vi "main.vi"() -> ()   [LabVIEW 2013]
uses:
  measure/Meas Session.ctl
  adc/ADC Session.ctl
  drivers/niScope/niScope Session.ctl
  drivers/niScope/niScope Virtual Channel Config.ctl
  drivers/niScope/niScope Virtual Channel Mode.ctl
  drivers/niScope/niScope Virtual Channel Input Z.ctl
  drivers/niScope/niScope Virtual Channel Coupling.ctl
  drivers/niScope/niScope Type.ctl
  drivers/niScope/niScope Digitizing Process Options.ctl
  drivers/niScope/niScope Data Packet.ctl
  drivers/niScope/niScope Trigger Setup.ctl
  <instrlib>/niScope/Controls/niScope trigger coupling.ctl
  <instrlib>/niScope/Controls/niScope trigger slope.ctl
  drivers/DMM/3458A Digitizer Session.ctl
  drivers/DMM/3458A Virtual Channel Config.ctl
  drivers/Counter/Counter Session.ctl
  drivers/Counter/Counter Type.ctl
  drivers/AWG/AWG Session.ctl
  drivers/AWG/AWG Type.ctl
  drivers/DMM/3458A Sync Mode.ctl
  drivers/DMM/3458A Idn Mode.ctl
  drivers/DMM/3458A Digitizing Low Levels/Configure/Sampling Mode.ctl
  drivers/DMM/3458A Digitizing Process Options.ctl
  drivers/DMM/3458A Data Packet.ctl
  drivers/DMM/3458A Aux Record Data.ctl
  drivers/DMM/3458A Digitizing Low Levels/Configure/Level Setup.ctl
  drivers/DMM/3458A Digitizing Low Levels/Configure/First Sample Trigger.ctl
  drivers/DMM/3458A Aperture Selection Mode.ctl
  drivers/dsdll/DSDLL Session.ctl
  drivers/dsdll/dsdll.lvlibp/dsdll_instance.ctl
  drivers/dsdll/dsdll.lvlibp/dsdll_device_record.ctl
  drivers/dsdll/DSDLL Process Config.ctl
  drivers/dsdll/DSDLL Data Packet.ctl
  adc/ADC Type.ctl
  drivers/simulated_adc/SimAdc Config.ctl
  drivers/simulated_adc/SimAdc Channel Cfg.ctl
  adc/ADC On Close Action.ctl
  drivers/Quatsch_driver/QuADCDriver/QuADC Session.ctl
  drivers/Quatsch_driver/QuADCDriver/QuADC Virtual Channel Config.ctl
  drivers/Quatsch_driver/QuADCDriver/QuADC Virtual Channel Mode.ctl
  drivers/Quatsch_driver/QuADCDriver/QuADC Virtual Channel Input Z.ctl
  drivers/Quatsch_driver/QuADCDriver/QuADC Virtual Channel Coupling.ctl
  drivers/Quatsch_driver/QuADCDriver/QuADC Type.ctl
  drivers/Quatsch_driver/QuADCDriver/QuADC Digitizing Process Options.ctl
  drivers/Quatsch_driver/QuADCDriver/QuADC Data Packet.ctl
  drivers/Quatsch_driver/QuADCDriver/QuADC Trigger Setup.ctl
  measure/Meas Sequence Item.ctl
  measure/Meas Sampling Configuration.ctl
  adc/ADC Trig Config.ctl
  adc/ADC Trig Mode Source.ctl
  adc/ADC Trig Coupling.ctl
  adc/ADC Trig Slope.ctl
  measure/processing/QWTB/Meas Proc QWTB Algorithm Parameter Data.ctl
  measure/Meas Sequence Configuration.ctl
  measure/Meas Range Mode.ctl
  measure/Meas Sampling Rate Mode.ctl
  octave/golpi/mpc/golpi_session_ref.ctl
  octave/golpi/mpc/golpi_session.ctl
  octave/golpi/GOLPI Library.lvlibp/Public/GOLPI reference Type Def.ctl
  octave/golpi/GOLPI Library.lvlibp/LV Process source distribution/Pipe Handle.ctl
  measure/processing/Meas Process Config.ctl
  measure/processing/Meas Process Mode.ctl
  measure/processing/Meas Process Raw Config.ctl
  measure/processing/Meas Process Raw Result Mode.ctl
  measure/processing/QWTB/Meas Proc QWTB Setup.ctl
  measure/processing/QWTB/Meas Proc QWTB Uncertainty Mode.ctl
  measure/processing/QWTB/Meas Proc QWTB Multicore Setup.ctl
  measure/processing/QWTB/Meas Proc QWTB Multicore Type.ctl
  measure/Corrections/Corr Setup.ctl
  measure/Corrections/Corr Tranducer Item.ctl
  measure/Corrections/Corr Digitizers.ctl
  measure/Assist/Assist Panel Setup.ctl
  measure/processing/QWTB/Meas Proc QWTB View Max Dim.ctl
  measure/processing/QWTB/Meas Proc QWTB View Uncertainty Mode.ctl
  measure/processing/QWTB/Meas Proc QWTB View Group Mode.ctl
  measure/processing/QWTB/Meas Proc QWTB Viewer References.ctl
  measure/processing/QWTB/Meas Proc QWTB View Phase Mode.ctl
  server/Server Event GUI command.ctl
  server/Server Session.ctl
  varilib/SGUI Assign References Mode.ctl
  server/Server Event.ctl
  server/Server Client Request.ctl
  server/Server Event Command.ctl
  <vilib>/Utility/miscctls.llb/LVRowAndColumnTypeDef.ctl
  varilib/SGUI Assign Multiple Strings With Tags By Label.vi
  varilib/varilib.lvlib
  drivers/niScope/niScope Virtual Digitizer.lvlib
  drivers/DMM/3458A Virtual Digitizer.lvlib
  drivers/Counter/Counter.lvlib
  drivers/AWG/AWG.lvlib
  drivers/DMM/3458A Digitizing Low Levels/3458A Digitizing Low Levels.lvlib
  drivers/dsdll/DSDLL Virtual Digitizer.lvlib
  drivers/dsdll/dsdll.lvlibp
  octave/golpi/mpc/GOLPI Multi Process.lvlib
  drivers/Quatsch_driver/QuADCDriver/QuADC Virtual Digitizer.lvlib
  octave/golpi/GOLPI Library.lvlibp/LV Process source distribution/LV Process library.lvlib
  octave/golpi/GOLPI Library.lvlibp
panel:
  in  "btn view fft":bool
  in  "server":T1
  out "start btns":T2
  in  "server vi ref":refnum<vi>
  in  "btn srv":bool
  in  "btn qwtb calc":bool
  in  "qwtb view VI ref":refnum<vi>
  in  "exp tab":string[][](table)
  in  "btn about":bool
  out "qwtb view":T3
  in  "tc result":enum32{"RAW", "QWTB"}(tab)
  out "str res":string caption="Result"
  out "qwtb meas pth":string caption="Selected measurement:"
  in  "qwtb alg sel":u16(ring) caption="Algorithm selection"
  in  "qwtb meas sel":u16(ring) caption="Measurement selection" items=["None", "Current", "Load from file"]
  in  "qwtb ref chn":u16(ring) caption="Ref. channel" items=["None"]
  in  "qwtb ph unit":T4 caption="Phase mode"
  out "qwtb res info":string caption="Info:"
  in  "qwtb res sel":u16(ring) caption="Result selection" items=["Current result", "Average"]
  in  "qwtb maxarr":i32=10 caption="Max shown array size" min=1 max=1000 step=1
  in  "qwtb order":T5 caption="Res. order mode"
  in  "qwtb unc":T6 caption="Uncertainty display"
  in  "qwtb maxdim":T7 caption="Max. shown dimension"
  out "qwtb results table":string[][](table) caption="Results (right click to table to show actions)"
  in  "qwtb qu list":i32[](listbox) caption="Select quantities"
  in  "btn set&start":bool
  in  "btn setup":bool
  in  "btn corr":bool
  in  "btn view rec":bool
  in  "golpi":T8={"GOLPI ref"={"pipe handle"={"lv_proc.dll file path"=path "", "process instance handle"=[], "debug mode"=FALSE, "debug data"=[]}, "fast read timeout [ms]"=500, "fast read settle time [ms]"=10, "fast read to multiple [ms]"=1, "max elements per input line"=100, "slow read timeout [ms]"=5000, "stdin double format specifier"="%_16e", "max elements per stdout output column"=100, "console mode bitstream"=FALSE, "bitstream first read timeout [ms]"=1000, "bitstream read timeout [ms]"=50, "struct transfer possible"=FALSE, "matlab mode"=FALSE}, "idn str"="", "octave path"=path "C:/Octave364/Octave3.6.4_gcc4.6.2/bin", "work path"=path "C:/Octave364/Octave3.6.4_gcc4.6.2/bin", "start timeout [ms]"=15000, "clr cache"=FALSE, "console"=FALSE, "binary"=FALSE, "semaphore"=refnum, "initial command"="", "exit command"="", "matlab"=FALSE}
  out "stat3":string
  out "stat2":string
  in  "session VI ref":refnum<vi>
  out "stat1":string
  in  "session":T12={"adc"={"niScope"={"channel cfg"=[], "sessions"=[], "multi cards"=FALSE, "channels"=0, "type"=enum."n/a", "memory [B/chn]"=0, "ext. clock [Hz]"=0.0, "samples count"=0, "use streaming"=FALSE, "proc setup"={"packet size [smpl]"=0, "current timeout [s]"=0.0, "blk2blk timeout [s]"=0.0, "event time"=timestamp(0 s since 1904-01-01), "temp sampl T [s]"=0.0, "data queue"=refnum, "stop notifier"=refnum, "proc ref"=refnum}, "sample width [B]"=0, "ranges [V]"=[], "trigger setup"={"coupling"=1, "level [V]"=0.0, "slope"=0, "mode"=enum."Immediate"}, "fs [Hz]"=0.0, "bitres [bit]"=0}, "3458A"={"channels"=[], "sync unit"={"VISA"="", "type"=enum."Picotest U6200A"}, "awg unit"={"type"=enum."Agilent 331xxA to 332xxA", "VISA"="", "enable 10MHz ref"=FALSE}, "sync mode"=enum."MASTER-SLAVE, MASTER clocked by TIMER", "streaming mode"=FALSE, "idn mode"=enum."Auto", "sampling mode"=enum."DCV", "Ts [s]"=0.0, "sample memory [B]"=0, "proc setup"={"channel id"=0, "packet size [smpl]"=0, "current timeout [s]"=0.0, "blk2blk timeout [s]"=0.0, "event time"=timestamp(0 s since 1904-01-01), "stop notifier"=refnum, "data queues"=[], "proc refs"=[], "bus semaphore"=refnum}, "sample size [B]"=0, "sample count"=0, "aux data"={"channel id"=0, "valid?"=[], "gain [V]"=[], "timestamp [s]"=[], "Ts [s]"=0.0, "abs timestamp"=timestamp(0 s since 1904-01-01), "t [deg C]"=[]}, "ranges [V]"=[], "aperture [s]"=0.0, "LEVEL trigger"={"edge"=enum."POS", "level [V]"=0.0, "coupling"=enum."DC"}, "trigger mode"=enum."AUTO", "measure temp.?"=FALSE, "disp mesages"=[], "shared bus?"=FALSE, "disable display?"=FALSE, "aper mode"=enum."Manual", "aper rules"=[]}, "dsdll"={"dsdll"={"dsdll path"=path "", "dsdll handle"=[], "output devices"=[], "capture devices"=[]}, "channels"=0, "device id"=0, "channel idns"=[], "proc setup"={"packet size [smpl]"=0, "current timeout [s]"=0.0, "blk2blk timeout [s]"=0.0, "event time"=timestamp(0 s since 1904-01-01), "data queue"=refnum, "stop notifier"=refnum, "proc ref"=refnum}, "samples count"=0, "fs [Hz]"=0.0}, "type"=enum."niScope", "channel idn str"=[], "aux instr idn str"=[], "modified?"=FALSE, "simadc"={"channels"=[], "range [V]"=0.0, "Ts step [s]"=0.0, "time [s]"=0.0, "fs [Hz]"=0.0, "count"=0, "smpl offset"=0, "set count"=0, "bit res"=0}, "force rst?"=FALSE, "exit mode"=enum."Immediate reset", "exit dly"=0.0, "exit tmr"=timestamp(0 s since 1904-01-01), "busy?"=FALSE, "accessed?"=FALSE, "QuADC session"={"channel cfg"=[], "sessions"=[], "multi cards"=FALSE, "channels"=0, "type"=enum."n/a", "memory [B/chn]"=0, "ext. clock [Hz]"=0.0, "samples count"=0, "use streaming"=FALSE, "proc setup"={"packet size [smpl]"=0, "current timeout [s]"=0.0, "blk2blk timeout [s]"=0.0, "event time"=timestamp(0 s since 1904-01-01), "temp sampl T [s]"=0.0, "data queue"=refnum, "stop notifier"=refnum, "proc ref"=refnum}, "sample width [B]"=0, "ranges [V]"=[], "trigger setup"={"coupling"=1, "level [V]"=0.0, "slope"=0, "mode"=enum."Immediate"}, "fs [Hz]"=0.0, "bitres [bit]"=0}}, "sequence"=[], "sequence setup"={"group setups"=[], "average cycles"=0, "range mode"=enum."Keep defaults", "fs mode"=enum."Frequency", "rng even"=0.0, "rng odd"=0.0, "folder"=path "", "name base"="", "meas id"=0, "settle [s]"=0.0}, "golpi"=refnum, "processing setup"={"mode"=enum."Raw", "call after avgs?"=FALSE, "calculate?"=FALSE, "raw mode"={"command"="", "result mode"=enum."Display console output (only Octave)", "res variable"=""}, "QWTB"={"QWTB path"=path "", "alg filter path"="", "alg ids"=[], "alg parameters"=[], "parsed parameters"=[], "selected alg id"="", "selected unc mode"=enum."None", "qwtb mcc"=100, "qwtb timeout"=90, "qwtb covg"=95.0, "qwtb ofs"=0, "qwtb lim data"=0, "multicore"={"jobs folder"=path "", "cores"=0, "max jobs"=0, "mode"=enum."Singlecore"}, "unc once?"=FALSE}}, "corrections"={"transducers"={"channels"=[], "last path"=path ""}, "digitizer"={"last path"=path "", "channel paths"=[], "channel idns"=[], "correction name"="", "channel names"=[], "folders to copy"=[], "channel valid"=[], "correction path"=path "", "correction rel path"="", "rel folders to copy"=[]}}, "assist cfg"={"P"=0, "Q"=0, "rel shift"=0.0, "ref freq"=0.0, "min fs"=0.0, "max fs tol"=0.0, "min int"=0.0, "max int"=0.0, "max err"=0.0, "max timeout"=0.0}} {"corrections"."transducers"."channels"."Phase index" min=1 step=1; "adc"."QuADC session"."trigger setup"."level [V]" format="%.2f"; "adc"."QuADC session"."trigger setup"."coupling" items=["AC"=0, "DC"=1, "HF Reject"=3, "LF Reject"=4, "AC Plus HF Reject"=1001]; "adc"."QuADC session"."channel cfg"."Clock fr. (Hz)" min=0.0 format="%#_9p"; "adc"."QuADC session"."channel cfg"."Number of JJ" min=1; "adc"."QuADC session"."channel cfg"."Range [Vpk]" min=0.0; "adc"."QuADC session"."channel cfg"."Channel" min=0; "adc"."3458A"."channels"."Range [Vpk]" min=0.0; "adc"."niScope"."trigger setup"."level [V]" format="%.2f"; "adc"."niScope"."trigger setup"."coupling" items=["AC"=0, "DC"=1, "HF Reject"=3, "LF Reject"=4, "AC Plus HF Reject"=1001]; "adc"."niScope"."channel cfg"."Range [Vpk]" min=0.0; "adc"."niScope"."channel cfg"."Channel" min=0}
  in  "btn stop":bool
  in  "btn start":bool
  out "error":errorcluster
  in  "btn exit":bool
  in  "btn cfg adc":bool
  in  "btn cfg octave":bool
  # "ADC:"
  # "IP Address"
  # "."
  # "."
  # "."
  # ":"
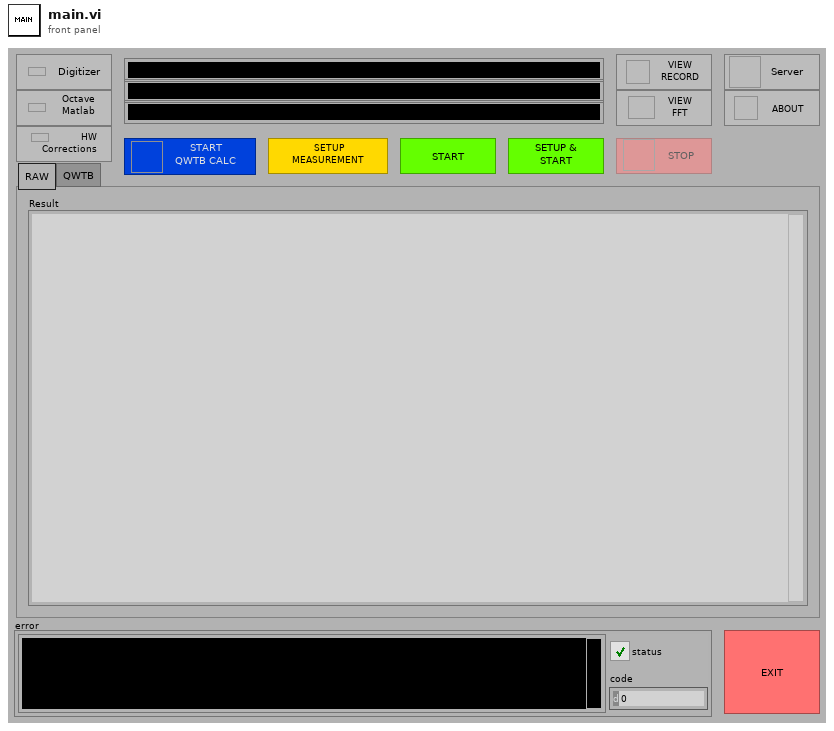
[diagram p1: front panel]
types:
  T1 = typedef "Server Session.ctl" = cluster{"cmd event":variant, "answer event":variant}
  T2 = typedef "Server Event GUI command.ctl" = cluster{"start":bool, "setup":bool, "setup&start":bool}
  T3 = typedef "Meas Proc QWTB Viewer References.ctl" = cluster{"tc result":refnum<vi>, "qwtb results tbl":refnum<vi>, "qwtb maxdim":refnum<vi>, "qwtb unc":refnum<vi>, "qwtb order":refnum<vi>, "qwtb maxarr":refnum<vi>, "qwtb res sel":refnum<vi>, "qwtb res info":refnum<vi>, "descriptions":string[], "var names":string[], "channel indexes":i32[], "qwtb ref chn":refnum<vi>, "qwtb ph unit":refnum<vi>, "qwtb alg sel":refnum<vi>, "qwtb meas sel":refnum<vi>, "qwtb ssn info":refnum<vi>, "last session":path, "qwtb qu list":refnum<vi>}
  T4 = typedef "Meas Proc QWTB View Phase Mode.ctl" = enum16{"± pi [rad]", "0 - 2*pi [rad]", "±180 [deg]", "0 - 360 [deg]"}
  T5 = typedef "Meas Proc QWTB View Group Mode.ctl" = enum16{"Group quantities", "Group phases"}
  T6 = typedef "Meas Proc QWTB View Uncertainty Mode.ctl" = enum16{"None", "val ± unc", "[val; unc]"}
  T7 = typedef "Meas Proc QWTB View Max Dim.ctl" = enum16{"Scalar", "Vector", "Matrix"}
  T8 = typedef "GOLPI Multi Process.lvlib/golpi_session.ctl" = cluster{"GOLPI ref":T9, "idn str":string, "octave path":path, "work path":path, "start timeout [ms]":u32, "clr cache":bool, "console":bool, "binary":bool, "semaphore":T11, "initial command":string, "exit command":string, "matlab":bool}
  T9 = typedef "GOLPI Library.lvlibp/GOLPI reference Type Def.ctl" = cluster{"pipe handle":T10, "fast read timeout [ms]":u32, "fast read settle time [ms]":u32, "fast read to multiple [ms]":u32, "max elements per input line":u32, "slow read timeout [ms]":u32, "stdin double format specifier":string, "max elements per stdout output column":u32, "console mode bitstream":bool, "bitstream first read timeout [ms]":u32, "bitstream read timeout [ms]":u32, "struct transfer possible":bool, "matlab mode":bool}
  T10 = typedef "GOLPI Library.lvlibp/LV Process library.lvlib/Pipe Handle.ctl" = cluster{"lv_proc.dll file path":path, "process instance handle":u32[], "debug mode":bool, "debug data":cluster{"time":timestamp, "stdin":bool, "data":string}[]}
  T11 = typedef "Semaphore RefNum" = refnum<k1>
  T12 = typedef "Meas Session.ctl" = cluster{"adc":T13, "sequence":T54[], "sequence setup":T61, "golpi":T64, "processing setup":T65, "corrections":T73, "assist cfg":T76}
  T13 = typedef "ADC Session.ctl" = cluster{"niScope":T14, "3458A":T24, "dsdll":T38, "type":T42, "channel idn str":string[], "aux instr idn str":string[], "modified?":bool, "simadc":T43, "force rst?":bool, "exit mode":T45, "exit dly":dbl, "exit tmr":timestamp, "busy?":bool, "accessed?":bool, "QuADC session":T46}
  T14 = typedef "niScope Virtual Digitizer.lvlib/niScope Session.ctl" = cluster{"channel cfg":T15[], "sessions":refnum<k20>[], "multi cards":bool, "channels":i32, "type":T19, "memory [B/chn]":i32, "ext. clock [Hz]":dbl, "samples count":i64, "use streaming":bool, "proc setup":T20, "sample width [B]":i32, "ranges [V]":dbl[], "trigger setup":T21, "fs [Hz]":dbl, "bitres [bit]":i32}
  T15 = typedef "niScope Virtual Digitizer.lvlib/niScope Virtual Channel Config.ctl" = cluster{"Address":refnum<k15>, "Channel":i32, "Mode":T16, "Input Z":T17, "Coupling":T18, "Range [Vpk]":dbl, "btn clr":bool, "btn up":bool, "btn down":bool}
  T16 = typedef "niScope Virtual Digitizer.lvlib/niScope Virtual Channel Mode.ctl" = enum16{"Single ended", "Unbal. differential", "Differential"}
  T17 = typedef "niScope Virtual Digitizer.lvlib/niScope Virtual Channel Input Z.ctl" = enum16{"1 MOhm", "50 Ohm"}
  T18 = typedef "niScope Virtual Digitizer.lvlib/niScope Virtual Channel Coupling.ctl" = enum16{"AC", "DC", "GND"}
  T19 = typedef "niScope Virtual Digitizer.lvlib/niScope Type.ctl" = enum16{"n/a", "5922"}
  T20 = typedef "niScope Virtual Digitizer.lvlib/niScope Digitizing Process Options.ctl" = cluster{"packet size [smpl]":i64, "current timeout [s]":dbl, "blk2blk timeout [s]":dbl, "event time":timestamp, "temp sampl T [s]":dbl, "data queue":refnum<queue>, "stop notifier":refnum<notifier>, "proc ref":refnum<vi>}
  T21 = typedef "niScope Virtual Digitizer.lvlib/niScope Trigger Setup.ctl" = cluster{"coupling":T22, "level [V]":dbl, "slope":T23, "mode":enum16{"Immediate", "External", "Level"}}
  T22 = typedef "niScope trigger coupling.ctl" = u16
  T23 = typedef "niScope trigger slope.ctl" = i32
  T24 = typedef "3458A Virtual Digitizer.lvlib/3458A Digitizer Session.ctl" = cluster{"channels":T25[], "sync unit":T26, "awg unit":T28, "sync mode":T30, "streaming mode":bool, "idn mode":T31, "sampling mode":T32, "Ts [s]":dbl, "sample memory [B]":i32, "proc setup":T33, "sample size [B]":i32, "sample count":i32, "aux data":T34, "ranges [V]":dbl[], "aperture [s]":dbl, "LEVEL trigger":T35, "trigger mode":T36, "measure temp.?":bool, "disp mesages":string[], "shared bus?":bool, "disable display?":bool, "aper mode":T37, "aper rules":dbl[][]}
  T25 = typedef "3458A Virtual Digitizer.lvlib/3458A Virtual Channel Config.ctl" = cluster{"VISA":refnum<visa-resource-name>, "Range [Vpk]":dbl, "btn clr":bool, "btn up":bool, "btn down":bool}
  T26 = typedef "Counter.lvlib/Counter Session.ctl" = cluster{"VISA":refnum<visa-resource-name>, "type":T27}
  T27 = typedef "Counter.lvlib/Counter Type.ctl" = enum16{"Picotest U6200A", "dummy"}
  T28 = typedef "AWG.lvlib/AWG Session.ctl" = cluster{"type":T29, "VISA":refnum<visa-resource-name>, "enable 10MHz ref":bool}
  T29 = typedef "AWG.lvlib/AWG Type.ctl" = enum16{"Agilent 331xxA to 332xxA", "Agilent 335xxA to 336xxA", "Tektronix AFG3101C", "dummy"}
  T30 = typedef "3458A Virtual Digitizer.lvlib/3458A Sync Mode.ctl" = enum16{"MASTER-SLAVE, MASTER clocked by TIMER", "MASTER-SLAVE, MASTER clocked by AWG", "ALL clocked by AWG", "MASTER-SLAVE, ALL clocked by TIMER", "ALL clocked by AWG with DFLL"}
  T31 = typedef "3458A Virtual Digitizer.lvlib/3458A Idn Mode.ctl" = enum16{"Auto", "Sequential (chn A, chn B, ...)", "From calibration string"}
  T32 = typedef "3458A Virtual Digitizer.lvlib/3458A Digitizing Low Levels.lvlib/Sampling Mode.ctl" = enum16{"DCV", "DSDC", "DSAC"}
  T33 = typedef "3458A Virtual Digitizer.lvlib/3458A Digitizing Process Options.ctl" = cluster{"channel id":i32, "packet size [smpl]":i32, "current timeout [s]":dbl, "blk2blk timeout [s]":dbl, "event time":timestamp, "stop notifier":refnum<notifier>, "data queues":refnum<queue>[], "proc refs":refnum<vi>[], "bus semaphore":T11}
  T34 = typedef "3458A Virtual Digitizer.lvlib/3458A Aux Record Data.ctl" = cluster{"channel id":i32, "valid?":bool[], "gain [V]":dbl[], "timestamp [s]":dbl[], "Ts [s]":dbl, "abs timestamp":timestamp, "t [deg C]":dbl[]}
  T35 = typedef "3458A Virtual Digitizer.lvlib/3458A Digitizing Low Levels.lvlib/Level Setup.ctl" = cluster{"edge":enum16{"POS", "NEG"}, "level [V]":dbl, "coupling":enum16{"DC", "AC"}}
  T36 = typedef "3458A Virtual Digitizer.lvlib/3458A Digitizing Low Levels.lvlib/First Sample Trigger.ctl" = enum16{"AUTO", "EXT", "SYN", "SGL", "HOLD", "LEVEL"}
  T37 = typedef "3458A Virtual Digitizer.lvlib/3458A Aperture Selection Mode.ctl" = enum16{"Manual", "Maximum", "Table"}
  T38 = typedef "DSDLL Virtual Digitizer.lvlib/DSDLL Session.ctl" = cluster{"dsdll":T39, "channels":i32, "device id":i32, "channel idns":string[], "proc setup":T41, "samples count":i32, "fs [Hz]":dbl}
  T39 = typedef "dsdll.lvlibp/dsdll_instance.ctl" = cluster{"dsdll path":path, "dsdll handle":u8[], "output devices":T40[], "capture devices":T40[]}
  T40 = typedef "dsdll.lvlibp/dsdll_device_record.ctl" = cluster{"guid":u8[], "name":string}
  T41 = typedef "DSDLL Virtual Digitizer.lvlib/DSDLL Process Config.ctl" = cluster{"packet size [smpl]":i32, "current timeout [s]":dbl, "blk2blk timeout [s]":dbl, "event time":timestamp, "data queue":refnum<queue>, "stop notifier":refnum<notifier>, "proc ref":refnum<vi>}
  T42 = typedef "ADC Type.ctl" = enum16{"niScope", "3458A", "DirectSound DLL", "dummy", "QuADC"}
  T43 = typedef "SimAdc Config.ctl" = cluster{"channels":T44[], "range [V]":dbl, "Ts step [s]":dbl, "time [s]":dbl, "fs [Hz]":dbl, "count":i64, "smpl offset":i64, "set count":i64, "bit res":i32}
  T44 = typedef "SimAdc Channel Cfg.ctl" = cluster{"harmonics":dbl[][], "btn clear":bool, "noise":dbl, "fundamental [Hz]":dbl}
  T45 = typedef "ADC On Close Action.ctl" = enum16{"Immediate reset", "Delayed reset"}
  T46 = typedef "QuADC Virtual Digitizer.lvlib/QuADC Session.ctl" = cluster{"channel cfg":T47[], "sessions":refnum<k5>[], "multi cards":bool, "channels":i32, "type":T51, "memory [B/chn]":i32, "ext. clock [Hz]":dbl, "samples count":i64, "use streaming":bool, "proc setup":T52, "sample width [B]":i32, "ranges [V]":dbl[], "trigger setup":T53, "fs [Hz]":dbl, "bitres [bit]":i32}
  T47 = typedef "QuADC Virtual Digitizer.lvlib/QuADC Virtual Channel Config.ctl" = cluster{"Channel":i32, "Mode":T48, "Input Z":T49, "Coupling":T50, "Range [Vpk]":dbl, "btn clr":bool, "btn up":bool, "btn down":bool, "IP address A":u8, "IP address B":u8, "IP address C":u8, "IP address D":u8, "Port":u16, "Number of JJ":u32, "Clock fr. (Hz)":dbl}
  T48 = typedef "QuADC Virtual Digitizer.lvlib/QuADC Virtual Channel Mode.ctl" = enum16{"Single ended", "Unbal. differential", "Differential"}
  T49 = typedef "QuADC Virtual Digitizer.lvlib/QuADC Virtual Channel Input Z.ctl" = enum16{"1 MOhm", "50 Ohm"}
  T50 = typedef "QuADC Virtual Digitizer.lvlib/QuADC Virtual Channel Coupling.ctl" = enum16{"AC", "DC", "GND"}
  T51 = typedef "QuADC Virtual Digitizer.lvlib/QuADC Type.ctl" = enum16{"n/a", "v1"}
  T52 = typedef "QuADC Virtual Digitizer.lvlib/QuADC Digitizing Process Options.ctl" = cluster{"packet size [smpl]":i64, "current timeout [s]":dbl, "blk2blk timeout [s]":dbl, "event time":timestamp, "temp sampl T [s]":dbl, "data queue":refnum<queue>, "stop notifier":refnum<notifier>, "proc ref":refnum<vi>}
  T53 = typedef "QuADC Virtual Digitizer.lvlib/QuADC Trigger Setup.ctl" = cluster{"coupling":T22, "level [V]":dbl, "slope":T23, "mode":enum16{"Immediate", "External", "Level"}}
  T54 = typedef "Meas Sequence Item.ctl" = cluster{"config":T55, "data file path":path, "header file path":path, "group id":i32, "average id":i32, "group done?":bool, "adc modified?":bool, "source modified?":bool, "progress [%]":dbl, "groups cnt":i32, "average cnt":i32, "data file relative path":string, "meas root path":path, "calculate?":bool}
  T55 = typedef "Meas Sampling Configuration.ctl" = cluster{"fs [Hz]":dbl, "count [smpl]":i64, "aperture [s]":dbl, "trigger":T56, "ranges [Vpk]":dbl[], "QWTB parameters":T60[]}
  T56 = typedef "ADC Trig Config.ctl" = cluster{"source":T57, "level [V]":dbl, "coupling":T58, "slope":T59}
  T57 = typedef "ADC Trig Mode Source.ctl" = enum16{"Immediate", "External", "Level"}
  T58 = typedef "ADC Trig Coupling.ctl" = enum16{"DC", "AC"}
  T59 = typedef "ADC Trig Slope.ctl" = enum16{"POS", "NEG"}
  T60 = typedef "Meas Proc QWTB Algorithm Parameter Data.ctl" = cluster{"name":string, "numerics":dbl[], "strings":string[]}
  T61 = typedef "Meas Sequence Configuration.ctl" = cluster{"group setups":T55[], "average cycles":i32, "range mode":T62, "fs mode":T63, "rng even":dbl, "rng odd":dbl, "folder":path, "name base":string, "meas id":i32, "settle [s]":dbl}
  T62 = typedef "Meas Range Mode.ctl" = enum16{"Keep defaults", "Set All channels", "Set Odd and Even channels"}
  T63 = typedef "Meas Sampling Rate Mode.ctl" = enum16{"Frequency", "Period"}
  T64 = typedef "GOLPI Multi Process.lvlib/golpi_session_ref.ctl" = refnum<vi>
  T65 = typedef "Meas Process Config.ctl" = cluster{"mode":T66, "call after avgs?":bool, "calculate?":bool, "raw mode":T67, "QWTB":T69}
  T66 = typedef "Meas Process Mode.ctl" = enum16{"Raw", "QWTB"}
  T67 = typedef "Meas Process Raw Config.ctl" = cluster{"command":string, "result mode":T68, "res variable":string}
  T68 = typedef "Meas Process Raw Result Mode.ctl" = enum16{"Display console output (only Octave)", "Display string variable", "Display result file %respath%"}
  T69 = typedef "Meas Proc QWTB Setup.ctl" = cluster{"QWTB path":path, "alg filter path":string, "alg ids":string[], "alg parameters":string[], "parsed parameters":T60[], "selected alg id":string, "selected unc mode":T70, "qwtb mcc":i32, "qwtb timeout":i32, "qwtb covg":dbl, "qwtb ofs":i64, "qwtb lim data":i64, "multicore":T71, "unc once?":bool}
  T70 = typedef "Meas Proc QWTB Uncertainty Mode.ctl" = enum16{"None", "GUF", "Monte Carlo"}
  T71 = typedef "Meas Proc QWTB Multicore Setup.ctl" = cluster{"jobs folder":path, "cores":i32, "max jobs":i32, "mode":T72}
  T72 = typedef "Meas Proc QWTB Multicore Type.ctl" = enum16{"Singlecore", "Multicore", "Multistation"}
  T73 = typedef "Corr Setup.ctl" = cluster{"transducers":cluster{"channels":T74[], "last path":path}, "digitizer":T75}
  T74 = typedef "Corr Tranducer Item.ctl" = cluster{"Path":path, "Ratio:":string, "Name:":string, "btn rem":bool, "btn up":bool, "btn down":bool, "s.n.:":string, "btn open":bool, "ratio o/i":dbl, "chn hi":u16, "chn lo":u16, "Phase index":i32}
  T75 = typedef "Corr Digitizers.ctl" = cluster{"last path":path, "channel paths":path[], "channel idns":string[], "correction name":string, "channel names":string[], "folders to copy":path[], "channel valid":bool[], "correction path":path, "correction rel path":string, "rel folders to copy":string[]}
  T76 = typedef "Assist Panel Setup.ctl" = cluster{"P":i32, "Q":i32, "rel shift":dbl, "ref freq":dbl, "min fs":dbl, "max fs tol":dbl, "min int":dbl, "max int":dbl, "max err":dbl, "max timeout":dbl}
  T77 = typedef "varilib.lvlib/SGUI Assign References Mode.ctl" = enum16{"Add to stack", "Overwrite", "Release last", "Release ID"}
  T78 = typedef "Server Event Command.ctl" = enum16{"None", "Restart", "Identify", "Set measurement", "Start", "Get status", "Get result", "Stop", "Set corrections", "Get algorithm info"}
  T79 = typedef "Server Event.ctl" = cluster{"client request":T80, "command":T78}
  T80 = typedef "Server Client Request.ctl" = cluster{"info data":string, "answer handle":i32}
  T81 = enum8{"Enabled", "Disabled", "Disabled and Grayed Out"}
  T82 = typedef "Meas Proc QWTB Plot Config.ctl" = cluster{"X-axis style":T83, "Y-axis style":T83, "Show legend":T84, "Grid on":bool, "Box on":bool, "show all chn":bool}
  T83 = typedef "Meas Proc QWTB Plot Scale Mode.ctl" = enum16{"Linear", "Log"}
  T84 = typedef "Meas Proc QWTB Plot Legend.ctl" = enum16{"None", "Best", "North", "South", "East", "West", "NorthEast", "NorthWest", "SouthEast", "SouthWest"}
  T85 = typedef "LVRowAndColumnTypeDef.ctl" = cluster{"Row":i32, "Column":i32}
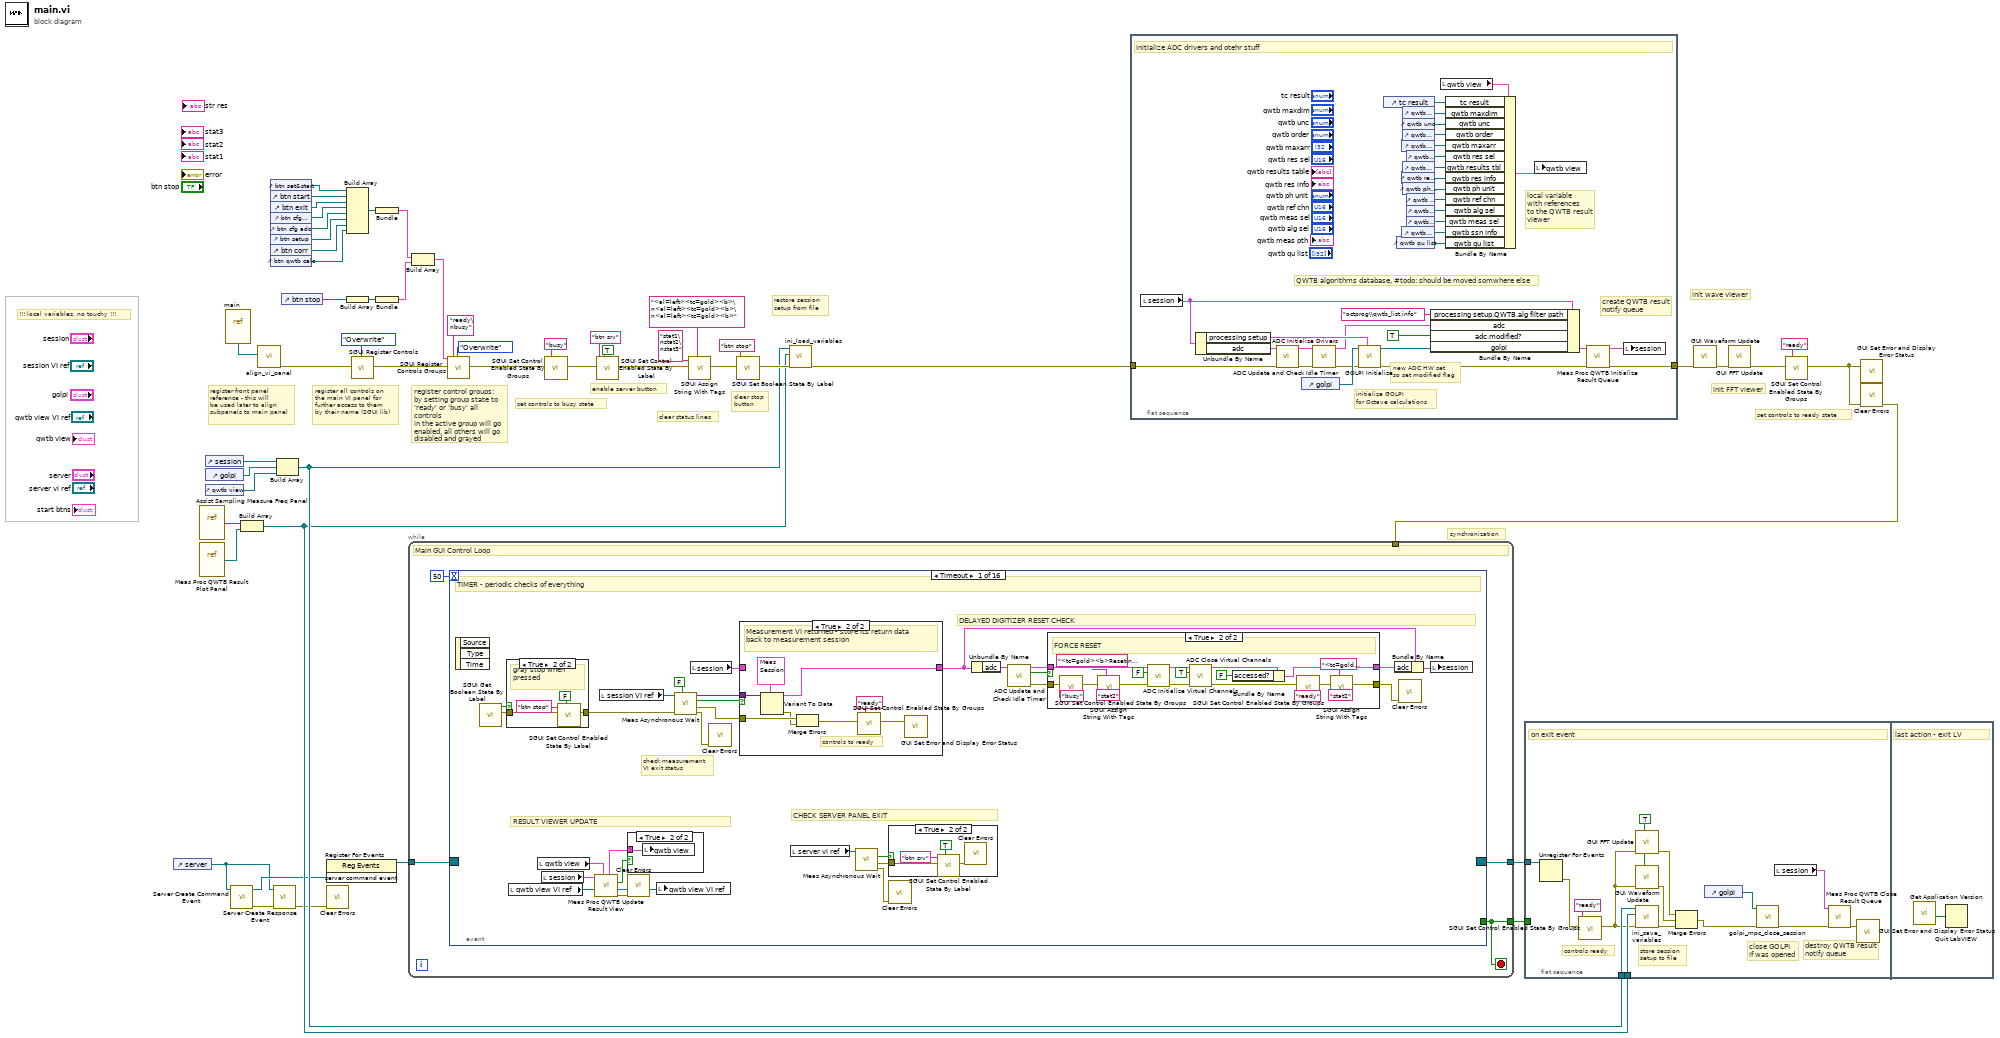
[diagram p0: block diagram]
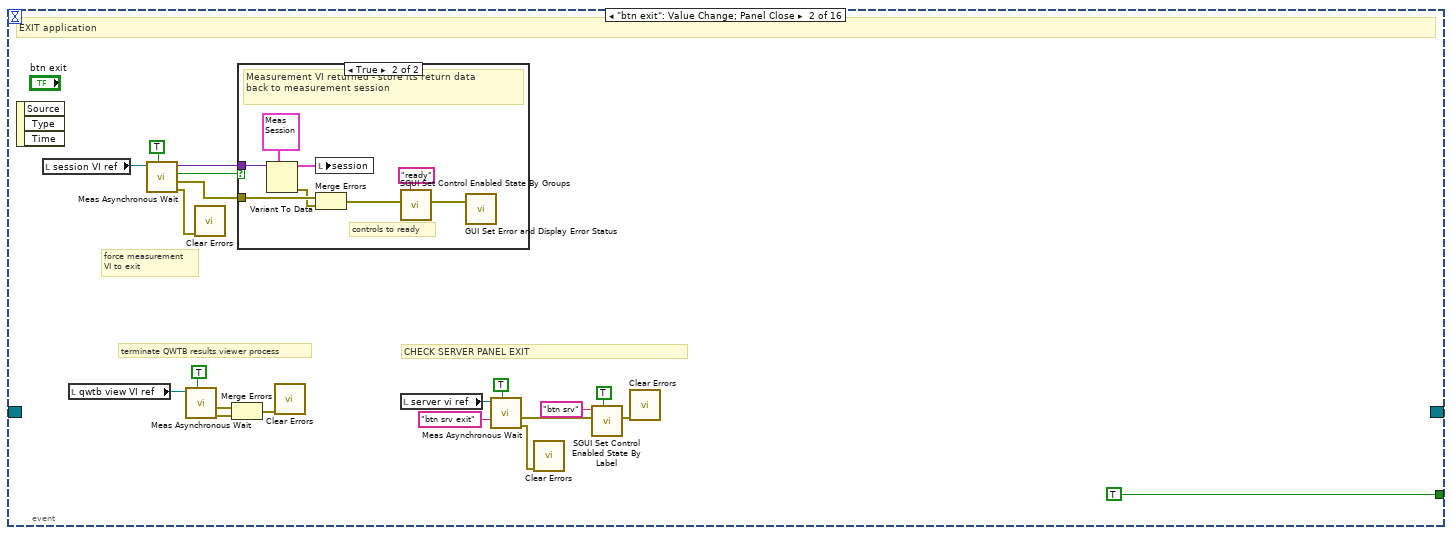
[diagram p7: hidden frame]
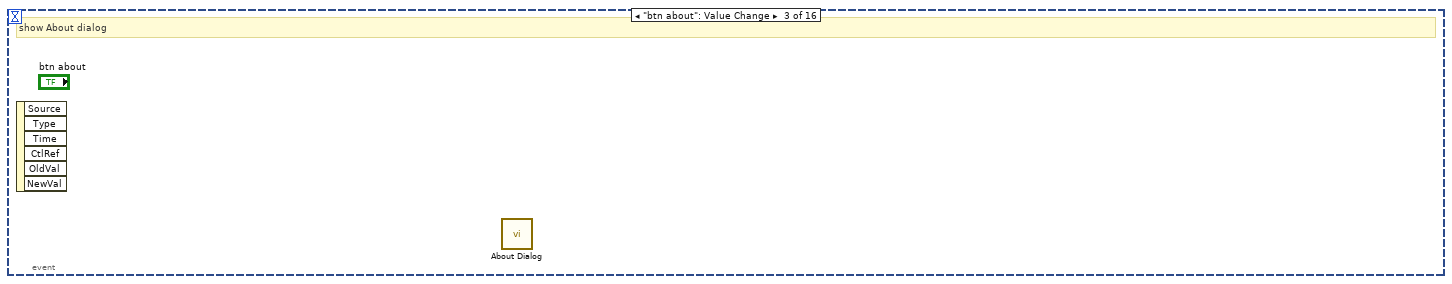
[diagram p9: hidden frame]
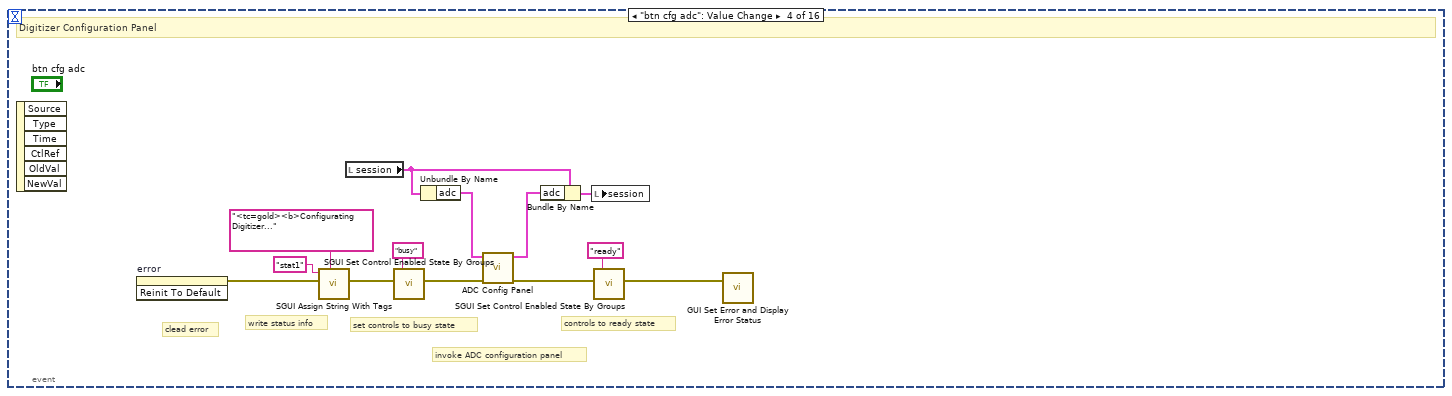
[diagram p10: hidden frame]
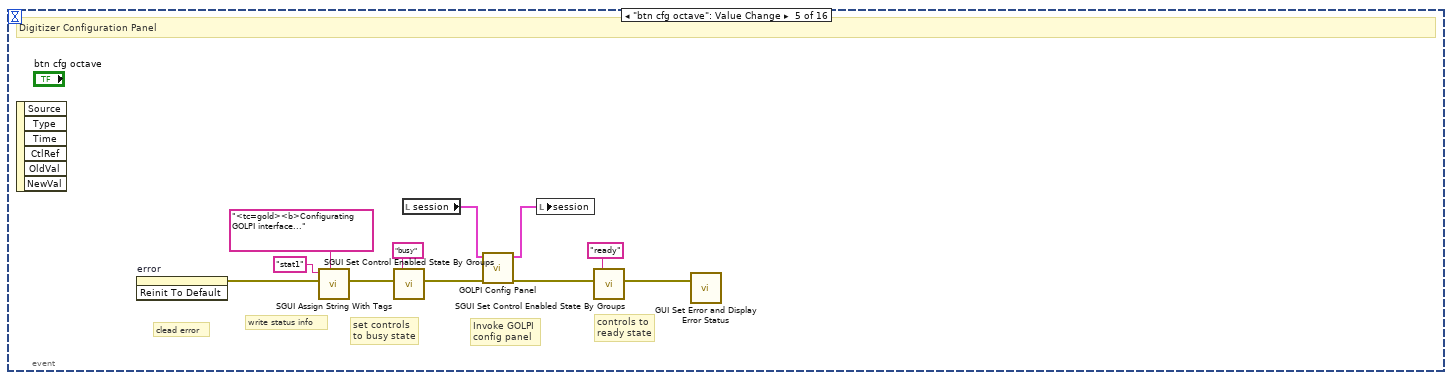
[diagram p11: hidden frame]
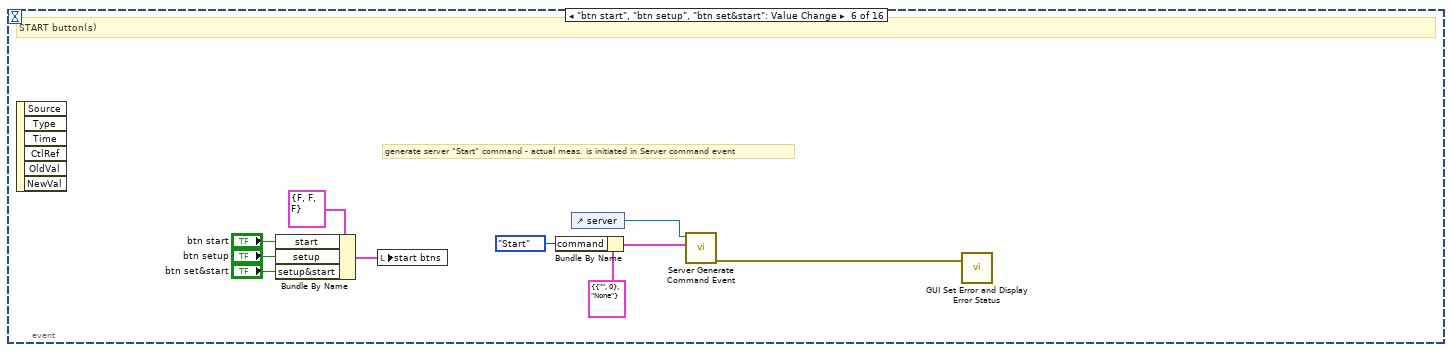
[diagram p12: hidden frame]
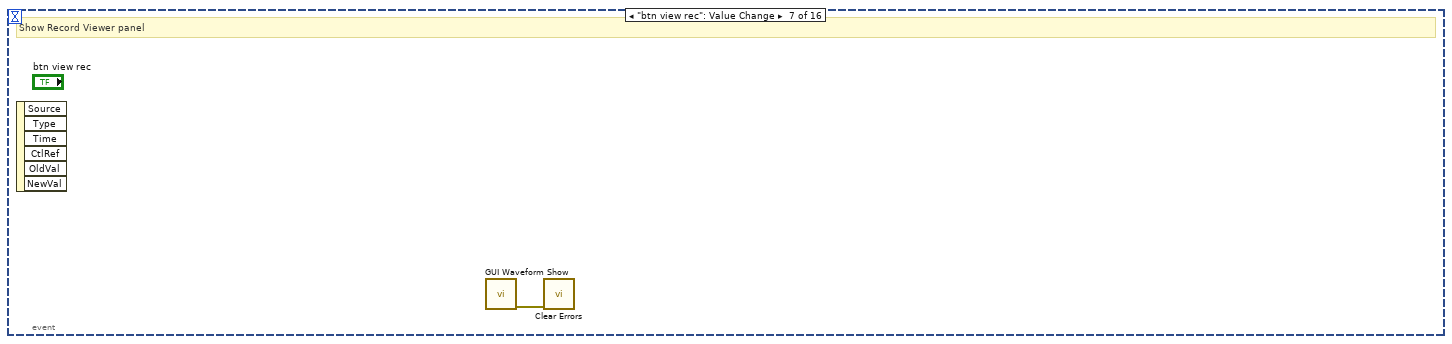
[diagram p13: hidden frame]
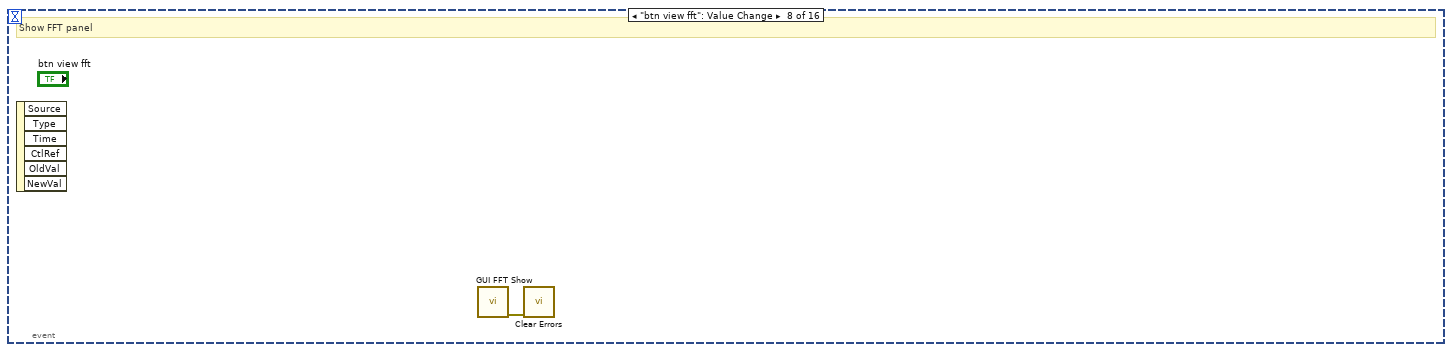
[diagram p14: hidden frame]
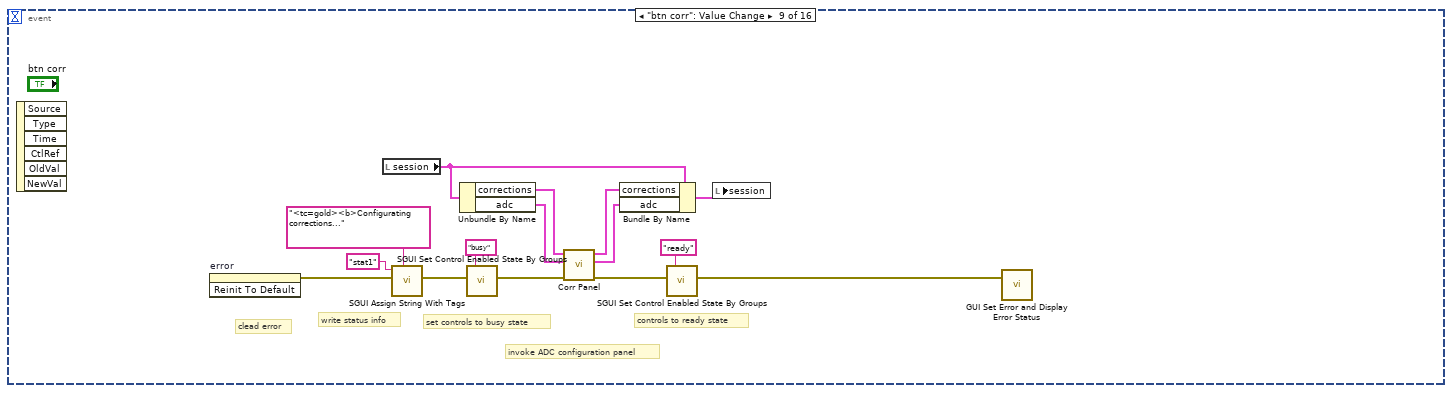
[diagram p15: hidden frame]
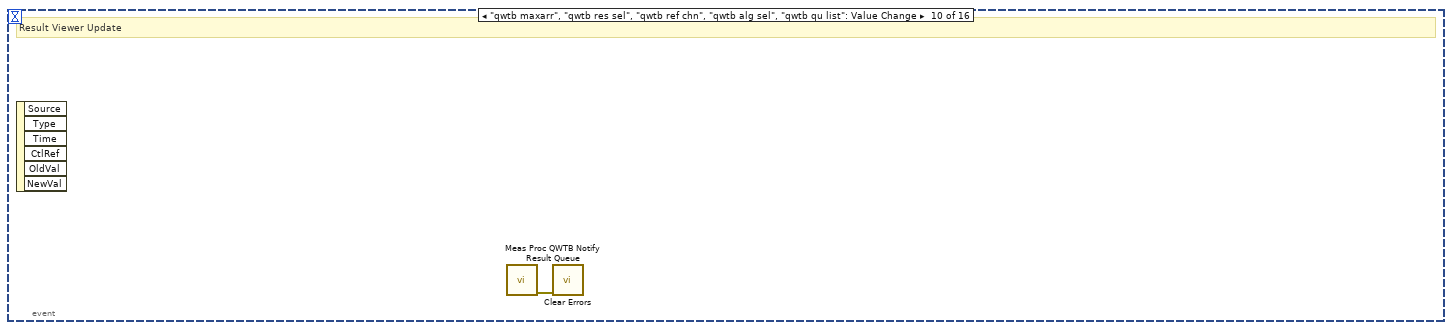
[diagram p16: hidden frame]
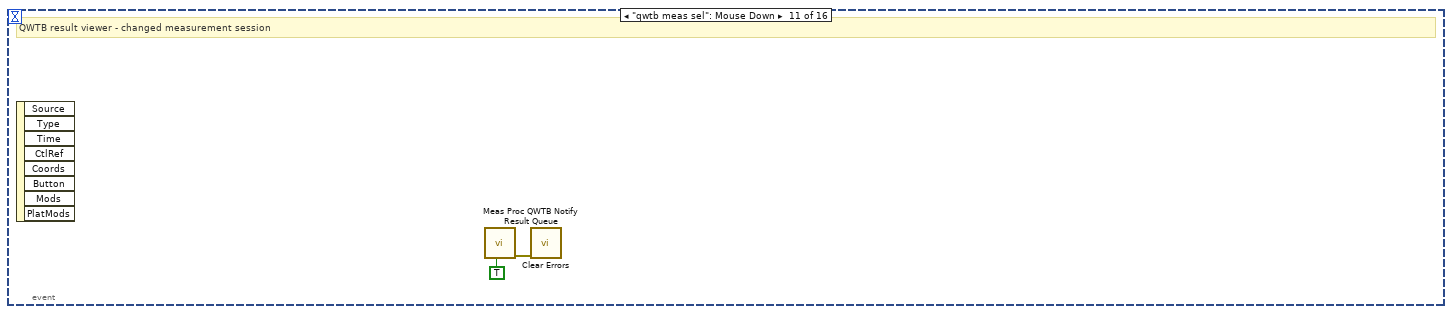
[diagram p17: hidden frame]
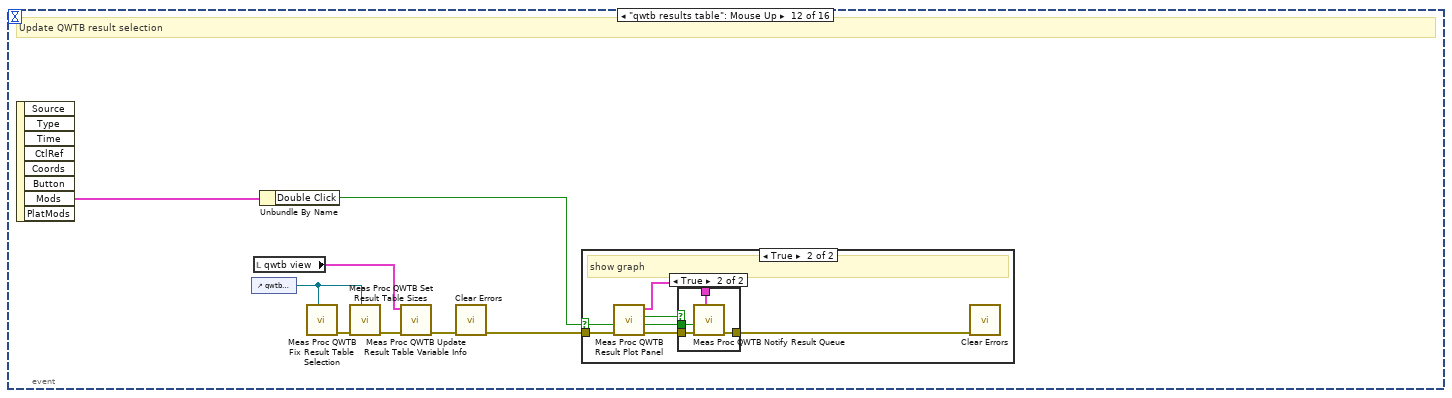
[diagram p18: hidden frame]
diagram:
  # "init FFT viewer"
  # "enable server button"
  # "init wave viewer"
  # "set controls to ready state"
  # "clear status lines"
  # "register front panel\nreference - this will\nbe used later to align\nsubpanels to main panel"
  # "restore session\nsetup from file"
  # "!!! local variables, no touchy !!!"
  # "clear stop\nbutton"
  # "synchronization"
  # "set controls to busy state"
  # "register control groups:\nby setting group state to\n'ready' or 'busy' all controls\nin the active group will go\nenabled, all others will go\ndisabled and grayed"
  # "register all controls on\nthe main VI panel for \nfurther access to them\nby their name (SGUI lib)"
  n1 = control-ref of="server"() -> (w7:refnum<vi>)
  n2 = vi-ref "Assist Sampling Measure Freq Panel.vi"() -> (w15:refnum<vi>)
  n3 = vi-ref "Meas Proc QWTB Result Plot Panel.vi"() -> (w13:refnum<vi>)
  n4 = control-ref of="session"() -> (w33:refnum<vi>)
  n5 = control-ref of="golpi"() -> (w28:refnum<vi>)
  n6 = control-ref of="qwtb view"() -> (w17:refnum<vi>)
  n7 = vi-ref "main.vi"() -> (w31:refnum<vi>)
  n8 = call "Server Create Command Event.vi"("server ref"=w7) -> ("error out"=w9:errorcluster, "server command event"=w11:refnum<user-event>)  [unwired: 9 in]
  n9 = Build Array(w15, w13) -> (w14:refnum<vi>[])
  n10 = call "align_vi_panel.vi"("top vi reference"=w31) -> ("error out"=w32:errorcluster)  [unwired: 10 in]
  n11 = control-ref of="btn set&start"() -> (w18:refnum<vi>)
  n12 = control-ref of="btn start"() -> (w47:refnum<vi>)
  n13 = control-ref of="btn exit"() -> (w46:refnum<vi>)
  n14 = control-ref of="btn cfg octave"() -> (w45:refnum<vi>)
  n15 = control-ref of="btn cfg adc"() -> (w44:refnum<vi>)
  n16 = control-ref of="btn setup"() -> (w20:refnum<vi>)
  n17 = control-ref of="btn corr"() -> (w19:refnum<vi>)
  n18 = control-ref of="btn qwtb calc"() -> (w16:refnum<vi>)
  n19 = call "Server Create Response Event.vi"("error in"=w9, "server ref"=w7) -> ("error out"=w8:errorcluster)  [unwired: 8 in, 1 out]
  n20 = Build Array(w33, w28, w17) -> (w24:refnum<vi>[])
  n21 = control-ref of="btn stop"() -> (w41:refnum<vi>)
  n22 = register-events(w11) -> (reference out=w12:refnum<event-registration>)  [unwired: 2 in, 1 out]
  n23 = call <vilib>:"Clear Errors.vi"("error in (no error)"=w8) -> ()  [unwired: 6 in, 1 out]
  n24 = Build Array(w18, w47, w46, w45, w44, w20, w19, w16) -> (w48:refnum<vi>[])
  n25 = Build Array(w41) -> (w42:refnum<vi>[])
  n26 = call "SGUI Register Controls.vi"("error in"=w32, "register mode (overwrite)"=SGUI_Assign_References_Mode."Overwrite") -> ("error out"=w51:errorcluster)  [unwired: 15 in, 2 out]
  n27 = Bundle(w48) -> (w49:cluster{refnum<vi>[]})  [unwired: 1 in]
  n28 = Bundle(w42) -> (w43:cluster{refnum<vi>[]})  [unwired: 1 in]
  n29 = Build Array(w49, w43) -> (w50:cluster{refnum<vi>[]}[])
  n30 = call "SGUI Register Controls Groups.vi"("control groups"=w50, "error in"=w51, "groups names"="ready\nbusy", "register mode (overwrite)"=SGUI_Assign_References_Mode."Overwrite") -> ("error out"=w38:errorcluster)  [unwired: 14 in, 1 out]
  n31 = call "SGUI Set Control Enabled State By Groups.vi"("error in"=w38, "group name to enable (none)"="busy") -> ("error out"=w6:errorcluster)  [unwired: 8 in, 1 out]
  n32 = call "SGUI Set Control Enabled State By Label.vi"("error in"=w6, "labels (empty)"="btn srv" ("control label(s) ('btn stop')"), "Enabled? (False)"=TRUE) -> ("error out"=w5:errorcluster)  [unwired: 7 in, 1 out]
  n33 = call-poly "SGUI Assign String With Tags.vi"("error in"=w5, "label(s) (empty)"="stat1\nstat2\nstat3", "string (empty)"="<al=left><tc=gold><b>\n<al=left><tc=gold><b>\n<al=left><tc=gold><b>") -> ("error out"=w27:errorcluster)  [unwired: 7 in, 1 out]
  n34 = call "SGUI Set Boolean State By Label.vi"("error in"=w27, "control label(s) ('btn stop')"="btn stop") -> ("error out"=w25:errorcluster)  [unwired: 8 in, 1 out]
  n35 = call "ini_load_variables.vi"("error in"=w25, "VI to store"=w14, "objects to store"=w24) -> ("error out"=w23:errorcluster)  [unwired: 8 in]
  n36 = flat-sequence {
    tunnel: w23 -> [w84]
    tunnel: [w76] -> w26
    frame #0 {
      # "local variable\nwith references\nto the QWTB result\nviewer"
      # "QWTB algorithms database, #todo: should be moved somwhere else"
      # "create QWTB result\nnotify queue"
      # "initialize GOLPI\nfor Octave calculations"
      # "new ADC HW set\nso set modified flag"
      # "initialize ADC drivers and otehr stuff"
      n37 = local read "session"() -> (w82:T12)
      n38 = Unbundle By Name(w82) -> ("processing setup"=w78:T65, "adc"=w83:T13)
      n39 = call "ADC Initialize Drivers.vi"("error in"=w84, "adc session in"=w83) -> ("error out"=w56:errorcluster, "adc session out"=w53:T13)  [unwired: 8 in]
      n40 = control-ref of="golpi"() -> (w79:refnum<vi>)
      n41 = call "ADC Update and Check Idle Timer.vi"("error in"=w56, "adc session in"=w53) -> ("error out"=w55:errorcluster, "adc session out"=w54:T13)  [unwired: 6 in, 2 out]
      n42 = call "GOLPI Initialize.vi"("processing setup"=w78, "error in"=w55, "golpi session ref"=w79) -> ("error out"=w77:errorcluster, "golpi session out (copy)"=w80:T64)  [unwired: 6 in, 1 out]
      n43 = control-ref of="tc result"() -> (w59:refnum<vi>)
      n44 = control-ref of="qwtb qu list"() -> (w57:refnum<vi>)
      n45 = control-ref of="qwtb maxarr"() -> (w63:refnum<vi>)
      n46 = control-ref of="qwtb res info"() -> (w66:refnum<vi>)
      n47 = control-ref of="qwtb meas pth"() -> (w71:refnum<vi>)
      n48 = control-ref of="qwtb maxdim"() -> (w60:refnum<vi>)
      n49 = control-ref of="qwtb unc"() -> (w61:refnum<vi>)
      n50 = control-ref of="qwtb order"() -> (w62:refnum<vi>)
      n51 = control-ref of="qwtb results table"() -> (w65:refnum<vi>)
      n52 = control-ref of="qwtb ph unit"() -> (w68:refnum<vi>)
      n53 = control-ref of="qwtb res sel"() -> (w64:refnum<vi>)
      n54 = control-ref of="qwtb ref chn"() -> (w67:refnum<vi>)
      n55 = control-ref of="qwtb alg sel"() -> (w69:refnum<vi>)
      n56 = control-ref of="qwtb meas sel"() -> (w70:refnum<vi>)
      n57 = Bundle By Name(cluster=w82, "processing setup.QWTB.alg filter path"="octprog\\qwtb_list.info", "adc"=w54, "adc.modified?"=TRUE, "golpi"=w80) -> (w75:T12)
      n58 = local read "qwtb view"() -> (w58:T3)
      n59 = Bundle By Name(cluster=w58, "tc result"=w59, "qwtb maxdim"=w60, "qwtb unc"=w61, "qwtb order"=w62, "qwtb maxarr"=w63, "qwtb res sel"=w64, "qwtb results tbl"=w65, "qwtb res info"=w66, "qwtb ph unit"=w68, "qwtb ref chn"=w67, "qwtb alg sel"=w69, "qwtb meas sel"=w70, "qwtb ssn info"=w71, "qwtb qu list"=w57) -> (w72:T3)
      n60 = local write "qwtb view"(w72) -> ()
      n61 = call "Meas Proc QWTB Initialize Result Queue.vi"("error in"=w77, "session in"=w75) -> ("error out"=w76:errorcluster, "session out"=w74:T12)  [unwired: 8 in]
      n62 = local write "session"(w74) -> ()
    }
  }
  n63 = flat-sequence {
    tunnel: w34 -> [_]
    tunnel: w24 -> [w98]
    tunnel: w14 -> [w94]
    tunnel: w10 -> [w93]
    frame #0 {
      w91 = TRUE ("Destroy notifier (False)")
      # "destroy QWTB result\nnotify queue"
      # "close GOLPI\nif was opened"
      # "store session\nsetup to file"
      # "controls ready"
      # "on exit event"
      n64 = Unregister For Events(event registration refnum=w93) -> (error out=w92:errorcluster)  [unwired: 1 in]
      n65 = call "SGUI Set Control Enabled State By Groups.vi"("error in"=w92, "group name to enable (none)"="ready") -> ("error out"=w90:errorcluster)  [unwired: 8 in, 1 out]
      n66 = call "GUI FFT Update.vi"("Destroy notifier (False)"=w91, "error in"=w90) -> ("error out"=w86:errorcluster)  [unwired: 9 in]
      n67 = call "GUI Waveform Update.vi"("Destroy notifier (False)"=w91, "error in"=w90) -> ("error out"=w87:errorcluster)  [unwired: 9 in]
      n68 = call "ini_save_variables.vi"("error in"=w90, "VI to store"=w94, "objects"=w98) -> ("error out"=w88:errorcluster)  [unwired: 8 in]
      n69 = Merge Errors(w86, w87, w88) -> (w85:errorcluster)
      n70 = control-ref of="golpi"() -> (w97:refnum<vi>)
      n71 = call "golpi_mpc_close_session.vi"("error in"=w85, "golpi session ref"=w97) -> ("error out"=w89:errorcluster)  [unwired: 8 in, 1 out]
      n72 = local read "session"() -> (w95:T12)
      n73 = call "Meas Proc QWTB Close Result Queue.vi"("error in"=w89, "session in"=w95) -> ("error out"=w96:errorcluster)  [unwired: 8 in, 1 out]
      n74 = call "GUI Set Error and Display Error Status.vi"("error in"=w96) -> ()  [unwired: 4 in]
    }
    frame #1 {
      # "last action - exit LV"
      n75 = call "Get Application Version.vi"() -> ("run time system"=w100:bool)  [unwired: 8 in, 3 out]
      n76 = Quit LabVIEW(quit? (T)=w100) -> ()
    }
  }
  n77 = call "GUI Waveform Update.vi"("error in"=w26) -> ("error out"=w2:errorcluster)  [unwired: 10 in]
  n78 = call "GUI FFT Update.vi"("error in"=w2) -> ("error out"=w1:errorcluster)  [unwired: 10 in]
  n79 = call "SGUI Set Control Enabled State By Groups.vi"("error in"=w1, "group name to enable (none)"="ready") -> ("error out"=w21:errorcluster)  [unwired: 8 in, 1 out]
  n80 = call "GUI Set Error and Display Error Status.vi"("error in"=w21) -> ()  [unwired: 4 in]
  n81 = call <vilib>:"Clear Errors.vi"("error in (no error)"=w21) -> ("error out"=w36:errorcluster)  [unwired: 6 in]
  n82 = while {
    tunnel: w36 -> [_]
    tunnel: [w103] -> w34
    tunnel: w12 -> [w102]
    tunnel: [w101] -> w10
    stop <- w103 stop-if-true
    # "Main GUI Control Loop"
    n83 = event shown="[0] Timeout" {
      selector: w102 -> [_ _ _ _ _ _ _ _ _ _ _ _ _ _ _ _]
      dyn-events: [_ _ _ _ _ _ _ _ _ _ _ _ _ _ _ _] -> w101
      timeout: 50 -> [_ _ _ _ _ _ _ _ _ _ _ _ _ _ _ _]
      tunnel: [_ TRUE _ _ _ _ _ _ _ _ _ _ _ _ _ _] -> w103
      event Timeout {
        # "DELAYED DIGITIZER RESET CHECK"
        # "CHECK SERVER PANEL EXIT"
        # "RESULT VIEWER UPDATE"
        # "check measurement\nVI exit status"
        # "TIMER - periodic checks of everything"
        n84 = event-data() -> ()  [unwired: 1 in, 3 out]
        n85 = call "SGUI Get Boolean State By Label.vi"() -> ("error out"=w127:errorcluster, "binary state out"=w126:bool)  [unwired: 9 in, 1 out]
        n86 = case shown="True" w126 {
          tunnel: w127 -> [w161 w165]
          tunnel: [w161 w163] -> w125
          frame False {
          }
          frame True {
            # "gray stop when\npressed"
            n87 = call "SGUI Set Control Enabled State By Label.vi"("error in"=w165, "labels (empty)"="btn stop", "Enabled? (False)"=FALSE) -> ("error out"=w163:errorcluster)  [unwired: 7 in, 1 out]
          }
        }
        n88 = local read "qwtb view VI ref"() -> (w119:refnum<vi>)
        n89 = local read "qwtb view"() -> (w123:T3)
        n90 = local read "session"() -> (w124:T12)
        n91 = call "Meas Proc QWTB Update Result View.vi"("QWTB result session in"=w123, "async VI reference in"=w119, "session in"=w124) -> ("error out"=w122:errorcluster, "async VI reference out"=w120:refnum<vi>, "VI returned?"=w118:bool, "QWTB result session out"=w121:T3)  [unwired: 4 in, 1 out]
        n92 = local read "session VI ref"() -> (w128:refnum<vi>)
        n93 = case shown="True" w118 {
          tunnel: w121 -> [_ w160]
          frame False {
          }
          frame True {
            n94 = local write "qwtb view"(w160) -> ()
          }
        }
        n95 = call <vilib>:"Clear Errors.vi"("error in (no error)"=w122) -> ()  [unwired: 6 in, 1 out]
        n96 = local write "qwtb view VI ref"(w120) -> ()
        n97 = call "Meas Asynchronous Wait.vi"("Wait for exit? (False)"=FALSE, "error in"=w125, "VI reference (empty)"=w128) -> ("error out"=w131:errorcluster, "VI's error out"=w132:errorcluster, "VI returned?"=w133:bool, "parameter out"=w129:variant)  [unwired: 4 in, 1 out]
        n98 = local read "session"() -> (w106:T12)
        n99 = call <vilib>:"Clear Errors.vi"("error in (no error)"=w131) -> ()  [unwired: 6 in, 1 out]
        n100 = case shown="True" w133 {
          tunnel: w132 -> [_ w172]
          tunnel: w129 -> [_ w174]
          tunnel: [w166 w167] -> w105
          tunnel: w106 -> [w166 _]
          frame False {
          }
          frame True {
            # "controls to ready"
            # "Measurement VI returned - store its return data\nback to measurement session"
            n101 = Variant To Data(type=T12 {"adc"={"niScope"={"channel cfg"=[], "sessions"=[], "multi cards"=FALSE, "channels"=0, "type"=enum."n/a", "memory [B/chn]"=0, "ext. clock [Hz]"=0.0, "samples count"=0, "use streaming"=FALSE, "proc setup"={"packet size [smpl]"=0, "current timeout [s]"=0.0, "blk2blk timeout [s]"=0.0, "event time"=timestamp(0 s since 1904-01-01), "temp sampl T [s]"=0.0, "data queue"=refnum, "stop notifier"=refnum, "proc ref"=refnum}, "sample width [B]"=0, "ranges [V]"=[], "trigger setup"={"coupling"=0, "level [V]"=0.0, "slope"=0, "mode"=enum."Immediate"}, "fs [Hz]"=0.0, "bitres [bit]"=0}, "3458A"={"channels"=[], "sync unit"={"VISA"="", "type"=enum."Picotest U6200A"}, "awg unit"={"type"=enum."Agilent 331xxA to 332xxA", "VISA"="", "enable 10MHz ref"=FALSE}, "sync mode"=enum."MASTER-SLAVE, MASTER clocked by TIMER", "streaming mode"=FALSE, "idn mode"=enum."Auto", "sampling mode"=enum."DCV", "Ts [s]"=0.0, "sample memory [B]"=0, "proc setup"={"channel id"=0, "packet size [smpl]"=0, "current timeout [s]"=0.0, "blk2blk timeout [s]"=0.0, "event time"=timestamp(0 s since 1904-01-01), "stop notifier"=refnum, "data queues"=[], "proc refs"=[], "bus semaphore"=refnum}, "sample size [B]"=0, "sample count"=0, "aux data"={"channel id"=0, "valid?"=[], "gain [V]"=[], "timestamp [s]"=[], "Ts [s]"=0.0, "abs timestamp"=timestamp(0 s since 1904-01-01), "t [deg C]"=[]}, "ranges [V]"=[], "aperture [s]"=0.0, "LEVEL trigger"={"edge"=enum."POS", "level [V]"=0.0, "coupling"=enum."DC"}, "trigger mode"=enum."AUTO", "measure temp.?"=FALSE, "disp mesages"=[], "shared bus?"=FALSE, "disable display?"=FALSE, "aper mode"=enum."Manual", "aper rules"=[]}, "dsdll"={"dsdll"={"dsdll path"=path "", "dsdll handle"=[], "output devices"=[], "capture devices"=[]}, "channels"=0, "device id"=0, "channel idns"=[], "proc setup"={"packet size [smpl]"=0, "current timeout [s]"=0.0, "blk2blk timeout [s]"=0.0, "event time"=timestamp(0 s since 1904-01-01), "data queue"=refnum, "stop notifier"=refnum, "proc ref"=refnum}, "samples count"=0, "fs [Hz]"=0.0}, "type"=enum."niScope", "channel idn str"=[], "aux instr idn str"=[], "modified?"=FALSE, "simadc"={"channels"=[], "range [V]"=0.0, "Ts step [s]"=0.0, "time [s]"=0.0, "fs [Hz]"=0.0, "count"=0, "smpl offset"=0, "set count"=0, "bit res"=0}, "force rst?"=FALSE, "exit mode"=enum."Immediate reset", "exit dly"=0.0, "exit tmr"=timestamp(0 s since 1904-01-01), "busy?"=FALSE, "accessed?"=FALSE, "QuADC session"={"channel cfg"=[], "sessions"=[], "multi cards"=FALSE, "channels"=0, "type"=enum."n/a", "memory [B/chn]"=0, "ext. clock [Hz]"=0.0, "samples count"=0, "use streaming"=FALSE, "proc setup"={"packet size [smpl]"=0, "current timeout [s]"=0.0, "blk2blk timeout [s]"=0.0, "event time"=timestamp(0 s since 1904-01-01), "temp sampl T [s]"=0.0, "data queue"=refnum, "stop notifier"=refnum, "proc ref"=refnum}, "sample width [B]"=0, "ranges [V]"=[], "trigger setup"={"coupling"=0, "level [V]"=0.0, "slope"=0, "mode"=enum."Immediate"}, "fs [Hz]"=0.0, "bitres [bit]"=0}}, "sequence"=[], "sequence setup"={"group setups"=[], "average cycles"=0, "range mode"=enum."Keep defaults", "fs mode"=enum."Frequency", "rng even"=0.0, "rng odd"=0.0, "folder"=path "", "name base"="", "meas id"=0, "settle [s]"=0.0}, "golpi"=refnum, "processing setup"={"mode"=enum."Raw", "call after avgs?"=FALSE, "calculate?"=FALSE, "raw mode"={"command"="", "result mode"=enum."Display console output (only Octave)", "res variable"=""}, "QWTB"={"QWTB path"=path "", "alg filter path"="", "alg ids"=[], "alg parameters"=[], "parsed parameters"=[], "selected alg id"="", "selected unc mode"=enum."None", "qwtb mcc"=0, "qwtb timeout"=0, "qwtb covg"=0.0, "qwtb ofs"=0, "qwtb lim data"=0, "multicore"={"jobs folder"=path "", "cores"=0, "max jobs"=0, "mode"=enum."Singlecore"}, "unc once?"=FALSE}}, "corrections"={"transducers"={"channels"=[], "last path"=path ""}, "digitizer"={"last path"=path "", "channel paths"=[], "channel idns"=[], "correction name"="", "channel names"=[], "folders to copy"=[], "channel valid"=[], "correction path"=path "", "correction rel path"="", "rel folders to copy"=[]}}, "assist cfg"={"P"=0, "Q"=0, "rel shift"=0.0, "ref freq"=0.0, "min fs"=0.0, "max fs tol"=0.0, "min int"=0.0, "max int"=0.0, "max err"=0.0, "max timeout"=0.0}} ("session"), Variant=w174) -> (data=w167:T12, error out=w171:errorcluster)  [unwired: 1 in]
            n102 = Merge Errors(w172, w171) -> (w170:errorcluster)
            n103 = call "SGUI Set Control Enabled State By Groups.vi"("error in"=w170, "group name to enable (none)"="ready") -> ("error out"=w169:errorcluster)  [unwired: 8 in, 1 out]
            n104 = call "GUI Set Error and Display Error Status.vi"("error in"=w169) -> ()  [unwired: 4 in]
          }
        }
        n105 = local read "server vi ref"() -> (w117:refnum<vi>)
        n106 = call "Meas Asynchronous Wait.vi"("VI reference (empty)"=w117) -> ("error out"=w114:errorcluster, "VI's error out"=w115:errorcluster, "VI returned?"=w116:bool)  [unwired: 6 in, 2 out]
        n107 = case shown="True" w116 {
          tunnel: w115 -> [_ w159]
          frame False {
          }
          frame True {
            n108 = call "SGUI Set Control Enabled State By Label.vi"("error in"=w159, "labels (empty)"="btn srv", "Enabled? (False)"=TRUE) -> ("error out"=w156:errorcluster)  [unwired: 7 in, 1 out]
            n109 = call <vilib>:"Clear Errors.vi"("error in (no error)"=w156) -> ()  [unwired: 6 in, 1 out]
          }
        }
        n110 = call <vilib>:"Clear Errors.vi"("error in (no error)"=w114) -> ()  [unwired: 6 in, 1 out]
        n111 = Unbundle By Name(w105) -> ("adc"=w113:T13)
        n112 = call "ADC Update and Check Idle Timer.vi"("adc session in"=w113) -> ("error out"=w111:errorcluster, "timeout?"=w110:bool, "adc session out"=w112:T13)  [unwired: 7 in, 1 out]
        n113 = case shown="True" w110 {
          tunnel: w112 -> [w134 w153]
          tunnel: w111 -> [w135 w146]
          tunnel: [w134 w150] -> w108
          tunnel: [w135 w136] -> w109
          frame False {
          }
          frame True {
            # "FORCE RESET"
            n114 = call "SGUI Set Control Enabled State By Groups.vi"("error in"=w146, "group name to enable (none)"="busy") -> ("error out"=w143:errorcluster)  [unwired: 8 in, 1 out]
            n115 = call-poly "SGUI Assign String With Tags.vi"("error in"=w143, "label(s) (empty)"="stat2", "string (empty)"="<tc=gold><b>Reseting digitizer to idle...") -> ("error out"=w142:errorcluster)  [unwired: 7 in, 1 out]
            n116 = call "ADC Initialize Virtual Channels.vi"("error in"=w142, "Reset? (False)"=FALSE, "adc session in"=w153) -> ("error out"=w155:errorcluster, "adc session out"=w154:T13)  [unwired: 4 in, 3 out]
            n117 = call "ADC Close Virtual Channels.vi"("error in"=w155, "Force reset to preset mode (False)"=TRUE, "adc session in"=w154) -> ("error out"=w144:errorcluster, "adc session out"=w149:T13)  [unwired: 7 in]
            n118 = Bundle By Name(cluster=w149, "accessed?"=FALSE) -> (w150:T13)
            n119 = call "SGUI Set Control Enabled State By Groups.vi"("error in"=w144, "group name to enable (none)"="ready") -> ("error out"=w137:errorcluster)  [unwired: 8 in, 1 out]
            n120 = call-poly "SGUI Assign String With Tags.vi"("error in"=w137, "label(s) (empty)"="stat2", "string (empty)"="<tc=gold><b>Digitizer was set to idle.") -> ("error out"=w136:errorcluster)  [unwired: 7 in, 1 out]
          }
        }
        n121 = Bundle By Name(cluster=w105, "adc"=w108) -> (w107:T12)
        n122 = call <vilib>:"Clear Errors.vi"("error in (no error)"=w109) -> ()  [unwired: 6 in, 1 out]
        n123 = local write "session"(w107) -> ()
      }
      event "btn exit": Value Change; Panel Close {
        # "CHECK SERVER PANEL EXIT"
        # "terminate QWTB results viewer process"
        # "force measurement\nVI to exit"
        # "EXIT application"
        n124 = event-data() -> ()  [unwired: 1 in, 3 out]
        n125 = local read "session VI ref"() -> (w188:refnum<vi>)
        n126 = local read "qwtb view VI ref"() -> (w183:refnum<vi>)
        n127 = call "Meas Asynchronous Wait.vi"("Wait for exit? (False)"=TRUE, "VI reference (empty)"=w188) -> ("error out"=w191:errorcluster, "VI's error out"=w192:errorcluster, "VI returned?"=w193:bool, "parameter out"=w189:variant)  [unwired: 5 in, 1 out]
        n128 = call "Meas Asynchronous Wait.vi"("Wait for exit? (False)"=TRUE, "VI reference (empty)"=w183) -> ("error out"=w185:errorcluster, "VI's error out"=w186:errorcluster)  [unwired: 5 in, 3 out]
        n129 = call <vilib>:"Clear Errors.vi"("error in (no error)"=w191) -> ()  [unwired: 6 in, 1 out]
        n130 = Merge Errors(w186, w185) -> (w184:errorcluster)
        n131 = case shown="True" w193 {
          tunnel: w192 -> [_ w200]
          tunnel: w189 -> [_ w202]
          frame False {
          }
          frame True {
            # "controls to ready"
            # "Measurement VI returned - store its return data\nback to measurement session"
            n132 = Variant To Data(type=T12 {"adc"={"niScope"={"channel cfg"=[], "sessions"=[], "multi cards"=FALSE, "channels"=0, "type"=enum."n/a", "memory [B/chn]"=0, "ext. clock [Hz]"=0.0, "samples count"=0, "use streaming"=FALSE, "proc setup"={"packet size [smpl]"=0, "current timeout [s]"=0.0, "blk2blk timeout [s]"=0.0, "event time"=timestamp(0 s since 1904-01-01), "temp sampl T [s]"=0.0, "data queue"=refnum, "stop notifier"=refnum, "proc ref"=refnum}, "sample width [B]"=0, "ranges [V]"=[], "trigger setup"={"coupling"=0, "level [V]"=0.0, "slope"=0, "mode"=enum."Immediate"}, "fs [Hz]"=0.0, "bitres [bit]"=0}, "3458A"={"channels"=[], "sync unit"={"VISA"="", "type"=enum."Picotest U6200A"}, "awg unit"={"type"=enum."Agilent 331xxA to 332xxA", "VISA"="", "enable 10MHz ref"=FALSE}, "sync mode"=enum."MASTER-SLAVE, MASTER clocked by TIMER", "streaming mode"=FALSE, "idn mode"=enum."Auto", "sampling mode"=enum."DCV", "Ts [s]"=0.0, "sample memory [B]"=0, "proc setup"={"channel id"=0, "packet size [smpl]"=0, "current timeout [s]"=0.0, "blk2blk timeout [s]"=0.0, "event time"=timestamp(0 s since 1904-01-01), "stop notifier"=refnum, "data queues"=[], "proc refs"=[], "bus semaphore"=refnum}, "sample size [B]"=0, "sample count"=0, "aux data"={"channel id"=0, "valid?"=[], "gain [V]"=[], "timestamp [s]"=[], "Ts [s]"=0.0, "abs timestamp"=timestamp(0 s since 1904-01-01), "t [deg C]"=[]}, "ranges [V]"=[], "aperture [s]"=0.0, "LEVEL trigger"={"edge"=enum."POS", "level [V]"=0.0, "coupling"=enum."DC"}, "trigger mode"=enum."AUTO", "measure temp.?"=FALSE, "disp mesages"=[], "shared bus?"=FALSE, "disable display?"=FALSE, "aper mode"=enum."Manual", "aper rules"=[]}, "dsdll"={"dsdll"={"dsdll path"=path "", "dsdll handle"=[], "output devices"=[], "capture devices"=[]}, "channels"=0, "device id"=0, "channel idns"=[], "proc setup"={"packet size [smpl]"=0, "current timeout [s]"=0.0, "blk2blk timeout [s]"=0.0, "event time"=timestamp(0 s since 1904-01-01), "data queue"=refnum, "stop notifier"=refnum, "proc ref"=refnum}, "samples count"=0, "fs [Hz]"=0.0}, "type"=enum."niScope", "channel idn str"=[], "aux instr idn str"=[], "modified?"=FALSE, "simadc"={"channels"=[], "range [V]"=0.0, "Ts step [s]"=0.0, "time [s]"=0.0, "fs [Hz]"=0.0, "count"=0, "smpl offset"=0, "set count"=0, "bit res"=0}, "force rst?"=FALSE, "exit mode"=enum."Immediate reset", "exit dly"=0.0, "exit tmr"=timestamp(0 s since 1904-01-01), "busy?"=FALSE, "accessed?"=FALSE, "QuADC session"={"channel cfg"=[], "sessions"=[], "multi cards"=FALSE, "channels"=0, "type"=enum."n/a", "memory [B/chn]"=0, "ext. clock [Hz]"=0.0, "samples count"=0, "use streaming"=FALSE, "proc setup"={"packet size [smpl]"=0, "current timeout [s]"=0.0, "blk2blk timeout [s]"=0.0, "event time"=timestamp(0 s since 1904-01-01), "temp sampl T [s]"=0.0, "data queue"=refnum, "stop notifier"=refnum, "proc ref"=refnum}, "sample width [B]"=0, "ranges [V]"=[], "trigger setup"={"coupling"=0, "level [V]"=0.0, "slope"=0, "mode"=enum."Immediate"}, "fs [Hz]"=0.0, "bitres [bit]"=0}}, "sequence"=[], "sequence setup"={"group setups"=[], "average cycles"=0, "range mode"=enum."Keep defaults", "fs mode"=enum."Frequency", "rng even"=0.0, "rng odd"=0.0, "folder"=path "", "name base"="", "meas id"=0, "settle [s]"=0.0}, "golpi"=refnum, "processing setup"={"mode"=enum."Raw", "call after avgs?"=FALSE, "calculate?"=FALSE, "raw mode"={"command"="", "result mode"=enum."Display console output (only Octave)", "res variable"=""}, "QWTB"={"QWTB path"=path "", "alg filter path"="", "alg ids"=[], "alg parameters"=[], "parsed parameters"=[], "selected alg id"="", "selected unc mode"=enum."None", "qwtb mcc"=0, "qwtb timeout"=0, "qwtb covg"=0.0, "qwtb ofs"=0, "qwtb lim data"=0, "multicore"={"jobs folder"=path "", "cores"=0, "max jobs"=0, "mode"=enum."Singlecore"}, "unc once?"=FALSE}}, "corrections"={"transducers"={"channels"=[], "last path"=path ""}, "digitizer"={"last path"=path "", "channel paths"=[], "channel idns"=[], "correction name"="", "channel names"=[], "folders to copy"=[], "channel valid"=[], "correction path"=path "", "correction rel path"="", "rel folders to copy"=[]}}, "assist cfg"={"P"=0, "Q"=0, "rel shift"=0.0, "ref freq"=0.0, "min fs"=0.0, "max fs tol"=0.0, "min int"=0.0, "max int"=0.0, "max err"=0.0, "max timeout"=0.0}} ("session"), Variant=w202) -> (data=w198:T12, error out=w199:errorcluster)  [unwired: 1 in]
            n133 = local write "session"(w198) -> ()
            n134 = Merge Errors(w200, w199) -> (w197:errorcluster)
            n135 = call "SGUI Set Control Enabled State By Groups.vi"("error in"=w197, "group name to enable (none)"="ready") -> ("error out"=w196:errorcluster)  [unwired: 8 in, 1 out]
            n136 = call "GUI Set Error and Display Error Status.vi"("error in"=w196) -> ()  [unwired: 4 in]
          }
        }
        n137 = call <vilib>:"Clear Errors.vi"("error in (no error)"=w184) -> ()  [unwired: 6 in, 1 out]
        n138 = local read "server vi ref"() -> (w182:refnum<vi>)
        n139 = call "Meas Asynchronous Wait.vi"("Wait for exit? (False)"=TRUE, "stop button name ('btn stop')"="btn srv exit", "VI reference (empty)"=w182) -> ("error out"=w180:errorcluster, "VI's error out"=w181:errorcluster)  [unwired: 4 in, 3 out]
        n140 = call <vilib>:"Clear Errors.vi"("error in (no error)"=w180) -> ()  [unwired: 6 in, 1 out]
        n141 = call "SGUI Set Control Enabled State By Label.vi"("error in"=w181, "labels (empty)"="btn srv", "Enabled? (False)"=TRUE) -> ("error out"=w175:errorcluster)  [unwired: 7 in, 1 out]
        n142 = call <vilib>:"Clear Errors.vi"("error in (no error)"=w175) -> ()  [unwired: 6 in, 1 out]
      }
      event "btn about": Value Change {
        # "show About dialog"
        n143 = event-data() -> ()  [unwired: 1 in, 6 out]
        n144 = call "About Dialog.vi"() -> ()  [unwired: 12 in]
      }
      event "btn cfg adc": Value Change {
        # "controls to ready state"
        # "clead error"
        # "write status info"
        # "set controls to busy state"
        # "invoke ADC configuration panel"
        # "Digitizer Configuration Panel"
        n145 = event-data() -> ()  [unwired: 1 in, 6 out]
        n146 = invoke on="error" class="Clust (strict)" method="Reinit To Default"() -> (error out=w207:errorcluster)  [unwired: 3 in, 2 out]
        n147 = call-poly "SGUI Assign String With Tags.vi"("error in"=w207, "label(s) (empty)"="stat1" ("control label (none)"), "string (empty)"="<tc=gold><b>Configurating Digitizer...") -> ("error out"=w206:errorcluster)  [unwired: 7 in, 1 out]
        n148 = local read "session"() -> (w214:T12)
        n149 = call "SGUI Set Control Enabled State By Groups.vi"("error in"=w206, "group name to enable (none)"="busy") -> ("error out"=w210:errorcluster)  [unwired: 8 in, 1 out]
        n150 = Unbundle By Name(w214) -> ("adc"=w215:T13)
        n151 = call "ADC Config Panel.vi"("error in"=w210, "adc session in"=w215) -> ("error out"=w208:errorcluster, "adc session out"=w213:T13)  [unwired: 8 in]
        n152 = Bundle By Name(cluster=w214, "adc"=w213) -> (w212:T12)
        n153 = local write "session"(w212) -> ()
        n154 = call "SGUI Set Control Enabled State By Groups.vi"("error in"=w208, "group name to enable (none)"="ready") -> ("error out"=w203:errorcluster)  [unwired: 8 in, 1 out]
        n155 = call "GUI Set Error and Display Error Status.vi"("error in"=w203) -> ()  [unwired: 4 in]
      }
      event "btn cfg octave": Value Change {
        # "controls to\nready state"
        # "clead error"
        # "write status info"
        # "set controls\nto busy state"
        # "Invoke GOLPI\nconfig panel"
        # "Digitizer Configuration Panel"
        n156 = event-data() -> ()  [unwired: 1 in, 6 out]
        n157 = invoke on="error" class="Clust (strict)" method="Reinit To Default"() -> (error out=w224:errorcluster)  [unwired: 3 in, 2 out]
        n158 = call-poly "SGUI Assign String With Tags.vi"("error in"=w224, "label(s) (empty)"="stat1" ("control label (none)"), "string (empty)"="<tc=gold><b>Configurating GOLPI interface...") -> ("error out"=w223:errorcluster)  [unwired: 7 in, 1 out]
        n159 = call "SGUI Set Control Enabled State By Groups.vi"("error in"=w223, "group name to enable (none)"="busy") -> ("error out"=w219:errorcluster)  [unwired: 8 in, 1 out]
        n160 = local read "session"() -> (w217:T12)
        n161 = call "GOLPI Config Panel.vi"("error in"=w219, "session in"=w217) -> ("error out"=w218:errorcluster, "session out"=w216:T12)  [unwired: 8 in]
        n162 = local write "session"(w216) -> ()
        n163 = call "SGUI Set Control Enabled State By Groups.vi"("error in"=w218, "group name to enable (none)"="ready") -> ("error out"=w220:errorcluster)  [unwired: 8 in, 1 out]
        n164 = call "GUI Set Error and Display Error Status.vi"("error in"=w220) -> ()  [unwired: 4 in]
      }
      event "btn start", "btn setup", "btn set&start": Value Change {
        # "generate server \"Start\" command - actual meas. is initiated in Server command event"
        # "START button(s)"
        n165 = event-data() -> ()  [unwired: 1 in, 6 out]
        n166 = Bundle By Name(cluster=T2 {"start"=FALSE, "setup"=FALSE, "setup&start"=FALSE} ("GUI request"), "start"="btn start", "setup"="btn setup", "setup&start"="btn set&start") -> (w228:T2)
        n167 = local write "start btns"(w228) -> ()
        n168 = Bundle By Name(cluster=T79 {"client request"={"info data"="", "answer handle"=0}, "command"=enum."None"} ("event data"), "command"=Server_Event_Command."Start") -> (w231:T79)
        n169 = control-ref of="server"() -> (w227:refnum<vi>)
        n170 = call "Server Generate Command Event.vi"("event data"=w231, "server event ref"=w227) -> ("error out"=w229:errorcluster)  [unwired: 9 in]
        n171 = call "GUI Set Error and Display Error Status.vi"("error in"=w229) -> ()  [unwired: 4 in]
      }
      event "btn view rec": Value Change {
        # "Show Record Viewer panel"
        n172 = event-data() -> ()  [unwired: 1 in, 6 out]
        n173 = call "GUI Waveform Show.vi"() -> ("error out"=w237:errorcluster)  [unwired: 11 in]
        n174 = call <vilib>:"Clear Errors.vi"("error in (no error)"=w237) -> ()  [unwired: 6 in, 1 out]
      }
      event "btn view fft": Value Change {
        # "Show FFT panel"
        n175 = event-data() -> ()  [unwired: 1 in, 6 out]
        n176 = call "GUI FFT Show.vi"() -> ("error out"=w238:errorcluster)  [unwired: 11 in]
        n177 = call <vilib>:"Clear Errors.vi"("error in (no error)"=w238) -> ()  [unwired: 6 in, 1 out]
      }
      event "btn corr": Value Change {
        # "controls to ready state"
        # "clead error"
        # "write status info"
        # "set controls to busy state"
        # "invoke ADC configuration panel"
        n178 = event-data() -> ()  [unwired: 1 in, 6 out]
        n179 = invoke on="error" class="Clust (strict)" method="Reinit To Default"() -> (error out=w247:errorcluster)  [unwired: 3 in, 2 out]
        n180 = local read "session"() -> (w253:T12)
        n181 = call-poly "SGUI Assign String With Tags.vi"("error in"=w247, "label(s) (empty)"="stat1" ("control label (none)"), "string (empty)"="<tc=gold><b>Configurating corrections...") -> ("error out"=w246:errorcluster)  [unwired: 7 in, 1 out]
        n182 = Unbundle By Name(w253) -> ("corrections"=w242:T73, "adc"=w240:T13)
        n183 = call "SGUI Set Control Enabled State By Groups.vi"("error in"=w246, "group name to enable (none)"="busy") -> ("error out"=w250:errorcluster)  [unwired: 8 in, 1 out]
        n184 = call "Corr Panel.vi"("error in"=w250, "adc session"=w240, "transducers in"=w242) -> ("error out"=w248:errorcluster, "adc session out"=w239:T13, "transducers out"=w241:T73)  [unwired: 6 in]
        n185 = Bundle By Name(cluster=w253, "corrections"=w241, "adc"=w239) -> (w252:T12)
        n186 = call "SGUI Set Control Enabled State By Groups.vi"("error in"=w248, "group name to enable (none)"="ready") -> ("error out"=w243:errorcluster)  [unwired: 8 in, 1 out]
        n187 = local write "session"(w252) -> ()
        n188 = call "GUI Set Error and Display Error Status.vi"("error in"=w243) -> ()  [unwired: 4 in]
      }
      event "qwtb maxarr", "qwtb res sel", "qwtb ref chn", "qwtb alg sel", "qwtb qu list": Value Change {
        # "Result Viewer Update"
        n189 = event-data() -> ()  [unwired: 1 in, 6 out]
        n190 = call "Meas Proc QWTB Notify Result Queue.vi"() -> ("error out"=w254:errorcluster)  [unwired: 10 in, 1 out]
        n191 = call <vilib>:"Clear Errors.vi"("error in (no error)"=w254) -> ()  [unwired: 6 in, 1 out]
      }
      event "qwtb meas sel": Mouse Down {
        # "QWTB result viewer - changed measurement session"
        n192 = event-data() -> ()  [unwired: 1 in, 8 out]
        n193 = call "Meas Proc QWTB Notify Result Queue.vi"("new session? (False)"=TRUE) -> ("error out"=w256:errorcluster)  [unwired: 9 in, 1 out]
        n194 = call <vilib>:"Clear Errors.vi"("error in (no error)"=w256) -> ()  [unwired: 6 in, 1 out]
      }
      event "qwtb results table": Mouse Up {
        # "Update QWTB result selection"
        n195 = event-data() -> ("Mods"=w264:cluster{"Double Click":bool, "Menu Key":bool})  [unwired: 1 in, 7 out]
        n196 = control-ref of="qwtb results table"() -> (w260:refnum<vi>)
        n197 = local read "qwtb view"() -> (w257:T3)
        n198 = Unbundle By Name(w264) -> ("Double Click"=w263:bool)
        n199 = call "Meas Proc QWTB Fix Result Table Selection.vi"("param table ref"=w260) -> ("error out"=w261:errorcluster)  [unwired: 10 in]
        n200 = call "Meas Proc QWTB Set Result Table Sizes.vi"("param table ref"=w260, "error in"=w261) -> ("error out"=w259:errorcluster)  [unwired: 9 in]
        n201 = call "Meas Proc QWTB Update Result Table Variable Info.vi"("error in"=w259, "QWTB result session in"=w257) -> ("error out"=w258:errorcluster)  [unwired: 9 in]
        n202 = call <vilib>:"Clear Errors.vi"("error in (no error)"=w258) -> ("error out"=w262:errorcluster)  [unwired: 6 in]
        n203 = case shown="True" w263 {
          selector: w263 -> [_ w269]
          tunnel: w262 -> [_ w266]
          frame False {
          }
          frame True {
            # "show graph"
            n204 = call "Meas Proc QWTB Result Plot Panel.vi"("error in"=w266) -> ("error out"=w268:errorcluster, "ok?"=w265:bool, "plot config"=w267:T82)  [unwired: 8 in]
            n205 = case shown="True" w265 {
              tunnel: [w271 w275] -> w270
              tunnel: w269 -> [_ w274]
              tunnel: w268 -> [w271 w273]
              tunnel: w267 -> [_ w272]
              frame False {
              }
              frame True {
                n206 = call "Meas Proc QWTB Notify Result Queue.vi"("plot setup"=w272, "error in"=w273, "show graph (False)"=w274) -> ("error out"=w275:errorcluster)  [unwired: 7 in, 1 out]
              }
            }
            n207 = call <vilib>:"Clear Errors.vi"("error in (no error)"=w270) -> ()  [unwired: 6 in, 1 out]
          }
        }
      }
      event "qwtb results table": Shortcut Menu Selection (User) {
        # "EXPORT QWTB RESULTS TABLE"
        n208 = event-data() -> ("ItemTag"=w276:string)  [unwired: 1 in, 7 out]
        n209 = case shown="Default" w276 {
          selector: w276 -> [_ _ _ w309]
          frame Default {
          }
          frame "QWTB_TAB_SHOW_GRAPH" {
            # "SHOW GRAPH"
            n210 = local read "qwtb view"() -> (w282:T3)
            n211 = call "Meas Proc QWTB Update Result Table Variable Info.vi"("QWTB result session in"=w282) -> ("error out"=w283:errorcluster)  [unwired: 10 in]
            n212 = call <vilib>:"Clear Errors.vi"("error in (no error)"=w283) -> ("error out"=w281:errorcluster)  [unwired: 6 in]
            n213 = call "Meas Proc QWTB Result Plot Panel.vi"("error in"=w281) -> ("error out"=w279:errorcluster, "ok?"=w277:bool, "plot config"=w278:T82)  [unwired: 8 in]
            n214 = case shown="True" w277 {
              tunnel: [w284 w288] -> w280
              tunnel: w279 -> [w284 w287]
              tunnel: w278 -> [_ w286]
              frame False {
              }
              frame True {
                n215 = call "Meas Proc QWTB Notify Result Queue.vi"("plot setup"=w286, "error in"=w287, "show graph (False)"=TRUE) -> ("error out"=w288:errorcluster)  [unwired: 7 in, 1 out]
              }
            }
            n216 = call <vilib>:"Clear Errors.vi"("error in (no error)"=w280) -> ()  [unwired: 6 in, 1 out]
          }
          frame "QWTB_TAB_CLOSE_GRAPHS" {
            # "Close all graphs"
            n217 = control-ref of="golpi"() -> (w291:refnum<vi>)
            n218 = call "golpi_mpc_get_access.vi"("golpi session ref"=w291) -> ("error out"=w296:errorcluster, "GOLPI ref out"=w294:T9, "golpi session ref out (copy)"=w292:T64)  [unwired: 5 in, 3 out]
            n219 = call "golpi_mpc_command.vi"("error in"=w296, "command"="close all;", "GOLPI ref in"=w294) -> ("error out"=w295:errorcluster, "GOLPI ref. out"=w293:T9)  [unwired: 6 in, 1 out]
            n220 = call "golpi_mpc_release.vi"("error in"=w295, "golpi ref or golpi session in"=w293, "golpi session ref"=w292) -> ("error out"=w289:errorcluster)  [unwired: 7 in, 1 out]
            n221 = call <vilib>:"Clear Errors.vi"("error in (no error)"=w289) -> ()  [unwired: 6 in, 1 out]
          }
          frame "QWTB_TAB_EXPORT_XLS", "QWTB_TAB_EXPORT_XLS_ROW" {
            w305 = T85 {"Row"=0, "Column"=0} ("Selection Start")
            # "build result table including headers, store to temp. matrix, export to Excel (this is needed in order ot export the headers with the data)"
            # "EXPORT TO EXCEL"
            n222 = property on="qwtb results table" class="Tbl (strict)"() -> (error out=w322:errorcluster, "Value"=w317:string[][], "Row Headers[]"=w316:string[], "Column Headers[]"=w315:string[])  [unwired: 2 in, 1 out]
            n223 = property on="qwtb results table" class="Tbl (strict)"() -> ("Selection Start"=w304:T85)  [unwired: 2 in, 2 out]
            n224 = Equal?(x="QWTB_TAB_EXPORT_XLS_ROW", y=w309) -> (x = y?=w302:bool)
            n225 = Transpose 2D Array(2D array=w317) -> (transposed array=w314:string[][])
            n226 = Unbundle By Name(w304) -> ("Row"=w303:i32)
            n227 = Build Array (concatenate)("", w315) -> (w312:string[])
            n228 = Build Array (concatenate)(w316, w314) -> (w323:string[][])
            n229 = Increment(x=w303) -> (x+1=w298:i32)
            n230 = Transpose 2D Array(2D array=w323) -> (transposed array=w313:string[][])
            n231 = Build Array (concatenate)(w312, w313) -> (w311:string[][])
            n232 = for {
              tunnel: [w324] -> w310 mode=indexing
              tunnel: w311 -> [w325] mode=indexing
              n233 = for {
                tunnel: [w328] -> w324 mode=indexing
                tunnel: w325 -> [w330] mode=indexing
                n234 = Empty String/Path?(string/path=w330) -> (empty?=w337:bool)
                n235 = Scan From String(format string="%.;%e", input string=w330) -> (error out=w327:errorcluster, output 1=w333:dbl)  [unwired: 3 in, 2 out]
                n236 = Scan From String(format string="%.;%p", input string=w330) -> (error out=w336:errorcluster, output 1=w332:dbl)  [unwired: 3 in, 2 out]
                n237 = Not Equal?(x=w333, y=w332) -> (x != y?=w326:bool)
                n238 = call <vilib>:"Clear Errors.vi"("error in (no error)"=w327) -> ()  [unwired: 6 in, 1 out]
                n239 = Compound Arithmetic op=AND(w326, invert w336, invert w337) -> (w335:bool)
                n240 = Format Into String(format string="%.;%_8g", w332) -> (resulting string=w331:string)  [unwired: 2 in, 1 out]
                n241 = Select(t=w331, s=w335, f=w330) -> (s? t:f=w328:string)
              }
            }
            n242 = property on="exp tab" class="Tbl (strict)"(error in=w322, "Value"=w310) -> (error out=w321:errorcluster)  [unwired: 1 in, 1 out]
            n243 = Array Size(array=w310) -> (size(s)=w320:i32[])
            n244 = Bundle By Name(cluster=w305, "Row"=w298) -> (w306:T85)
            n245 = Array To Cluster(array=w320) -> (cluster=w299:cluster{"[0]":i32, "[1]":i32})
            n246 = Bundle By Name(cluster=w299, "[0]"=1) -> (w300:cluster{"[0]":i32, "[1]":i32})
            n247 = Select(t=w306, s=w302, f=w305) -> (s? t:f=w307:T85)
            n248 = Select(t=w300, s=w302, f=w299) -> (s? t:f=w301:cluster{"[0]":i32, "[1]":i32})
            n249 = property on="exp tab" class="Tbl (strict)"(error in=w321, "Selection Start"=w307, "Selection Size"=w301) -> (error out=w319:errorcluster)  [unwired: 1 in, 1 out]
            n250 = invoke on="exp tab" class="Tbl (strict)" method="Export Data to Excel"(error in=w319) -> ()  [unwired: 2 in, 3 out]
          }
        }
      }
      event "btn qwtb calc": Value Change {
        # "controls to ready state"
        # "clead error"
        # "write status info"
        # "set controls to busy state"
        # "invoke ADC configuration panel"
        # "Run QWTB batch processing panel"
        n251 = event-data() -> ()  [unwired: 1 in, 6 out]
        n252 = invoke on="error" class="Clust (strict)" method="Reinit To Default"() -> (error out=w347:errorcluster)  [unwired: 3 in, 2 out]
        n253 = call-poly "SGUI Assign String With Tags.vi"("error in"=w347, "label(s) (empty)"="stat1" ("control label (none)"), "string (empty)"="<tc=gold><b>QWTB batch processing...") -> ("error out"=w346:errorcluster)  [unwired: 7 in, 1 out]
        n254 = call "SGUI Set Control Enabled State By Groups.vi"("error in"=w346, "group name to enable (none)"="busy") -> ("error out"=w342:errorcluster)  [unwired: 8 in, 1 out]
        n255 = local read "session"() -> (w340:T12)
        n256 = call "Meas Batch Proc QWTB Panel.vi"("error in"=w342, "session in"=w340) -> ("error out"=w341:errorcluster, "session out"=w339:T12)  [unwired: 8 in]
        n257 = local write "session"(w339) -> ()
        n258 = call "SGUI Set Control Enabled State By Groups.vi"("error in"=w341, "group name to enable (none)"="ready") -> ("error out"=w343:errorcluster)  [unwired: 8 in, 1 out]
        n259 = call "GUI Set Error and Display Error Status.vi"("error in"=w343) -> ()  [unwired: 4 in]
      }
      event "btn srv": Value Change {
        # "Start TWM server"
        n260 = event-data() -> ()  [unwired: 1 in, 6 out]
        n261 = invoke on="error" class="Clust (strict)" method="Reinit To Default"() -> (error out=w352:errorcluster)  [unwired: 3 in, 2 out]
        n262 = control-ref of="server"() -> (w351:refnum<vi>)
        n263 = vi-ref "Server Panel.vi"() -> (w354:refnum<vi>)
        n264 = To Variant(anything=w351) -> (Variant=w355:variant)
        n265 = call "Meas Asynchronous Start.vi"("error in"=w352, "parameter in"=w355, "Static VI reference in (empty)"=w354) -> ("error out"=w350:errorcluster, "async VI reference out"=w353:refnum<vi>)  [unwired: 7 in]
        n266 = local write "server vi ref"(w353) -> ()
        n267 = call "GUI Set Error and Display Error Status.vi"("error in"=w350) -> ()  [unwired: 4 in]
        n268 = case shown="No Error" w350 {
          frame No Error {
            n269 = call "SGUI Set Control Enabled State By Label.vi"("labels (empty)"="btn srv", "Enabled? (False)"=FALSE) -> ()  [unwired: 8 in, 2 out]
          }
          frame Error {
          }
        }
      }
      event User Event {
        # "SERVER COMMANDS EVENT HANDLER"
        n270 = event-data() -> ("client request"=w360:T80, "command"=w361:T78)  [unwired: 1 in, 4 out]
        n271 = property on="btn stop" class="Bool (strict)"() -> (error out=w359:errorcluster, "DisabledEnum"=w358:T81)  [unwired: 2 in, 1 out]
        n272 = case shown="\"Start\"" w361 {
          tunnel: w360 -> [_ w364 _ _ _ _ w474 w503 w520]
          tunnel: w359 -> [_ w363 w384 w437 w456 w462 w472 w501 w518]
          tunnel: w358 -> [_ w362 w385 w436 w457 w463 w473 w502 w519]
          frame Default {
          }
          frame "Set measurement" {
            n273 = case shown="\"Disabled and Grayed Out\"" w362 {
              tunnel: w364 -> [_ w373]
              tunnel: w363 -> [_ w365]
              frame Default {
              }
              frame "Disabled and Grayed Out" {
                # "send ACK"
                # "no GUI"
                # "parse and set\nsampling and\nprocessing parameters"
                # "controls ready"
                # "invoke config panel or config\nvalidity check\n\nnote: here in server mode\nit will just regenerate sequence\nand check destination path"
                # "update status"
                # "controls busy"
                n274 = invoke on="error" class="Clust (strict)" method="Reinit To Default"(error in=w365) -> (error out=w379:errorcluster)  [unwired: 2 in, 2 out]
                n275 = call-poly "SGUI Assign String With Tags.vi"("error in"=w379, "label(s) (empty)"="stat1\nstat2\nstat3", "string (empty)"="<tc=gold><b>TWM server - Setting new measurement...\n\n") -> ("error out"=w378:errorcluster)  [unwired: 7 in, 1 out]
                n276 = call "SGUI Set Control Enabled State By Groups.vi"("error in"=w378, "group name to enable (none)"="busy") -> ("error out"=w376:errorcluster)  [unwired: 8 in, 1 out]
                n277 = local read "session"() -> (w375:T12)
                n278 = call "Server Cmd Parser - Set Measurement.vi"("error in"=w376, "client request"=w373, "session in"=w375) -> ("error out"=w374:errorcluster, "session out"=w367:T12)  [unwired: 7 in]
                n279 = call "Meas Config Panel.vi"("error in"=w374, "force no GUI (False)"=TRUE, "session in"=w367) -> ("error out"=w371:errorcluster, "session out"=w366:T12)  [unwired: 6 in, 1 out]
                n280 = local write "session"(w366) -> ()
                n281 = control-ref of="server"() -> (w369:refnum<vi>)
                n282 = call "Server Generate ACK Event.vi"("error in"=w371, "header"="Set measurement" ("event data"), "server event ref"=w369) -> ("error out"=w370:errorcluster)  [unwired: 8 in]
                n283 = call "SGUI Set Control Enabled State By Groups.vi"("error in"=w370, "group name to enable (none)"="ready") -> ("error out"=w381:errorcluster)  [unwired: 8 in, 1 out]
                n284 = call "GUI Set Error and Display Error Status.vi"("error in"=w381) -> ()  [unwired: 4 in]
              }
            }
          }
          frame "Start" {
            n285 = case shown="\"Disabled and Grayed Out\"" w385 {
              tunnel: w384 -> [_ w387]
              frame Default {
              }
              frame "Disabled and Grayed Out" {
                # "server command?"
                # "invoke config\npanel or config\nvalidity check"
                # "start measurement"
                # "update status"
                # "controls busy"
                n286 = local read "start btns"() -> (w396:T2)
                n287 = Unbundle By Name(w396) -> ("start"=w395:bool, "setup"=w394:bool, "setup&start"=w393:bool)
                n288 = invoke on="error" class="Clust (strict)" method="Reinit To Default"(error in=w387) -> (error out=w408:errorcluster)  [unwired: 2 in, 2 out]
                n289 = Compound Arithmetic op=OR(w393, w394, w395) -> (invert w390:bool)
                n290 = flat-sequence {
                  tunnel: w390 -> [_]
                  frame #0 {
                    n291 = local write "start btns"(T2 {"start"=FALSE, "setup"=FALSE, "setup&start"=FALSE} ("start btns")) -> ()
                  }
                }
                n292 = call-poly "SGUI Assign String With Tags.vi"("error in"=w408, "label(s) (empty)"="stat1\nstat2\nstat3", "string (empty)"="<tc=gold><b>Starting measurement...\n\n") -> ("error out"=w407:errorcluster)  [unwired: 7 in, 1 out]
                n293 = call "SGUI Set Control Enabled State By Groups.vi"("error in"=w407, "group name to enable (none)"="busy") -> ("error out"=w404:errorcluster)  [unwired: 8 in, 1 out]
                n294 = local read "session"() -> (w389:T12)
                n295 = Compound Arithmetic op=OR(w394, w393) -> (w398:bool)
                n296 = call "Meas Config Panel.vi"("error in"=w404, "force no GUI (False)"=w390, "always show setup (False)"=w398, "session in"=w389) -> ("error out"=w403:errorcluster, "canceled?"=w400:bool, "session out"=w388:T12)  [unwired: 5 in]
                n297 = Compound Arithmetic op=OR(w390, w395, w393) -> (w397:bool)
                n298 = Compound Arithmetic op=AND(w397, invert w400) -> (invert w399:bool)
                n299 = case shown="False" w399 {
                  tunnel: [w426 _] -> w405
                  tunnel: w403 -> [w423 w429]
                  tunnel: w388 -> [w422 w428]
                  tunnel: [w425 w429] -> w401
                  tunnel: [w418 w428] -> w386
                  frame False {
                    # "digitizer busy"
                    n300 = Unbundle By Name(w422) -> ("adc"=w424:T13)
                    n301 = call "ADC Reset Idle Timer.vi"("error in"=w423, "set busy (False)"=TRUE, "adc session in"=w424) -> ("error out"=w420:errorcluster, "adc session out"=w421:T13)  [unwired: 7 in]
                    n302 = Bundle By Name(cluster=w422, "adc"=w421) -> (w418:T12)
                    n303 = vi-ref "Meas Main.vi"() -> (w427:refnum<vi>)
                    n304 = call "Meas Asynchronous Start.vi"("error in"=w420, "parameter in"=w418, "Static VI reference in (empty)"=w427) -> ("error out"=w425:errorcluster, "async VI reference out"=w426:refnum<vi>)  [unwired: 7 in]
                  }
                  frame True {
                  }
                }
                n305 = local write "session"(w386) -> ()
                n306 = Compound Arithmetic op=OR(w401, w399) -> (w402:bool)
                n307 = case shown="True" w402 {
                  tunnel: [w431 w434] -> w392
                  tunnel: [TRUE _] -> w410
                  tunnel: w405 -> [w432 _]
                  tunnel: w401 -> [w431 w433]
                  frame False {
                    # "success, remember\nsession VI reference"
                    n308 = local write "session VI ref"(w432) -> ()
                  }
                  frame True {
                    # "controls ready"
                    # "async start failed\nrestore controls"
                    n309 = call "SGUI Set Control Enabled State By Groups.vi"("error in"=w433, "group name to enable (none)"="ready") -> ("error out"=w434:errorcluster)  [unwired: 8 in, 1 out]
                  }
                }
                n310 = case shown="True" w390 {
                  tunnel: w392 -> [w413 w414]
                  tunnel: [w413 w416] -> w391
                  frame False {
                  }
                  frame True {
                    # "Server ACK"
                    n311 = control-ref of="server"() -> (w417:refnum<vi>)
                    n312 = call "Server Generate ACK Event.vi"("error in"=w414, "header"="Start", "server event ref"=w417) -> ("error out"=w416:errorcluster)  [unwired: 8 in]
                  }
                }
                n313 = call "GUI Set Error and Display Error Status.vi"("error in"=w391, "Write status only if error occures? (False)"=w410) -> ()  [unwired: 3 in]
              }
            }
          }
          frame "Identify" {
            n314 = case shown="\"Disabled and Grayed Out\"" w436 {
              tunnel: w437 -> [_ w438]
              frame Default {
              }
              frame "Disabled and Grayed Out" {
                # "identify instruments"
                # "controls ready"
                # "update status"
                # "controls busy"
                n315 = invoke on="error" class="Clust (strict)" method="Reinit To Default"(error in=w438) -> (error out=w451:errorcluster)  [unwired: 2 in, 2 out]
                n316 = call-poly "SGUI Assign String With Tags.vi"("error in"=w451, "label(s) (empty)"="stat1\nstat2\nstat3", "string (empty)"="<tc=gold><b>TWM server - Identification of instruments...\n\n") -> ("error out"=w450:errorcluster)  [unwired: 7 in, 1 out]
                n317 = call "SGUI Set Control Enabled State By Groups.vi"("error in"=w450, "group name to enable (none)"="busy") -> ("error out"=w448:errorcluster)  [unwired: 8 in, 1 out]
                n318 = local read "session"() -> (w446:T12)
                n319 = Unbundle By Name(w446) -> ("adc"=w447:T13)
                n320 = call "ADC Get Capabilities.vi"("Initialize HW? (False)"=TRUE, "error in"=w448, "adc session in"=w447) -> ("error out"=w443:errorcluster, "adc session out"=w441:T13)  [unwired: 6 in, 1 out]
                n321 = Bundle By Name(cluster=w446, "adc"=w441) -> (w445:T12)
                n322 = local write "session"(w445) -> ()
                n323 = control-ref of="server"() -> (w442:refnum<vi>)
                n324 = call "Server Cmd Answer - Identify.vi"("server event ref"=w442, "error in"=w443, "command header (none)"="Identify", "adc session"=w441) -> ("error out"=w444:errorcluster)  [unwired: 6 in, 1 out]
                n325 = call "SGUI Set Control Enabled State By Groups.vi"("error in"=w444, "group name to enable (none)"="ready") -> ("error out"=w453:errorcluster)  [unwired: 8 in, 1 out]
                n326 = call "GUI Set Error and Display Error Status.vi"("error in"=w453) -> ()  [unwired: 4 in]
              }
            }
          }
          frame "Get status" {
            # "is ready?"
            n327 = Equal?(x=w457, y=T81."Disabled and Grayed Out") -> (x = y?=w458:bool)
            n328 = control-ref of="server"() -> (w459:refnum<vi>)
            n329 = call "Server Cmd Answer - Get Status.vi"("server event ref"=w459, "error in"=w456, "Status ready? (False)"=w458) -> ("error out"=w460:errorcluster)  [unwired: 7 in, 1 out]
            n330 = call <vilib>:"Clear Errors.vi"("error in (no error)"=w460) -> ()  [unwired: 6 in, 1 out]
          }
          frame "Stop" {
            # "send ACK"
            # "Set STOP state if running"
            n331 = case shown="\"Enabled\"" w463 {
              tunnel: w462 -> [w468 w470]
              tunnel: [w468 w469] -> w467
              frame Default {
              }
              frame "Enabled" {
                n332 = property on="btn stop" class="Bool (strict)"(error in=w470, "Val(Sgnl)"=TRUE ("Value (Signaling)")) -> (error out=w469:errorcluster)  [unwired: 1 in, 1 out]
              }
            }
            n333 = control-ref of="server"() -> (w466:refnum<vi>)
            n334 = call "Server Generate ACK Event.vi"("error in"=w467, "header"="Stop", "server event ref"=w466) -> ("error out"=w464:errorcluster)  [unwired: 8 in]
            n335 = call <vilib>:"Clear Errors.vi"("error in (no error)"=w464) -> ()  [unwired: 6 in, 1 out]
          }
          frame "Set corrections" {
            n336 = case shown="\"Disabled and Grayed Out\"" w473 {
              tunnel: w474 -> [_ w499]
              tunnel: w472 -> [_ w479]
              frame Default {
              }
              frame "Disabled and Grayed Out" {
                w494 = "" ("status name label")
                # "send ACK"
                # "update status"
                # "controls busy"
                n337 = invoke on="error" class="Clust (strict)" method="Reinit To Default"(error in=w479) -> (error out=w485:errorcluster)  [unwired: 2 in, 2 out]
                n338 = call-poly "SGUI Assign String With Tags.vi"("error in"=w485, "label(s) (empty)"="stat1\nstat2\nstat3", "string (empty)"="<tc=gold><b>TWM server - Setting corrections...\n\n") -> ("error out"=w484:errorcluster)  [unwired: 7 in, 1 out]
                n339 = call "SGUI Set Control Enabled State By Groups.vi"("error in"=w484, "group name to enable (none)"="busy") -> ("error out"=w482:errorcluster)  [unwired: 8 in, 1 out]
                n340 = local read "session"() -> (w500:T12)
                n341 = call "Server Cmd Parser - Set Corrections.vi"("error in"=w482, "client request"=w499, "session in"=w500) -> ("error out"=w495:errorcluster, "session out"=w491:T12)  [unwired: 7 in]
                n342 = Unbundle By Name(w491) -> ("corrections.transducers"=w498:cluster{"channels":T74[], "last path":path}, "corrections.digitizer"=w497:T75, "adc"=w496:T13)
                n343 = call "Corr Transducers Reload All.vi"("error in"=w495, "transducers in"=w498) -> ("error out"=w493:errorcluster, "transducers out"=w490:cluster{"channels":T74[], "last path":path})  [unwired: 8 in]
                n344 = call "Corr Digitizer Check.vi"("correction path label"=w494, "status name label"=w494, "correction name label"=w494, "error in"=w495, "adc session"=w496, "digitizer corrections in"=w497) -> ("error out"=w492:errorcluster, "digitizer corrections out"=w489:T75)  [unwired: 2 in, 2 out]
                n345 = Bundle By Name(cluster=w491, "corrections.transducers"=w490, "corrections.digitizer"=w489) -> (w488:T12)
                n346 = Merge Errors(w493, w492) -> (w476:errorcluster)
                n347 = local write "session"(w488) -> ()
                n348 = control-ref of="server"() -> (w478:refnum<vi>)
                n349 = call "Server Generate ACK Event.vi"("error in"=w476, "header"="Set corrections" ("event data"), "server event ref"=w478) -> ("error out"=w475:errorcluster)  [unwired: 8 in]
                n350 = call "SGUI Set Control Enabled State By Groups.vi"("error in"=w475, "group name to enable (none)"="ready") -> ("error out"=w480:errorcluster)  [unwired: 8 in, 1 out]
                n351 = call "GUI Set Error and Display Error Status.vi"("error in"=w480) -> ()  [unwired: 4 in]
              }
            }
          }
          frame "Get result" {
            n352 = case shown="\"Disabled and Grayed Out\"" w502 {
              tunnel: w503 -> [_ w507]
              tunnel: w501 -> [_ w504]
              frame Default {
              }
              frame "Disabled and Grayed Out" {
                n353 = invoke on="error" class="Clust (strict)" method="Reinit To Default"(error in=w504) -> (error out=w515:errorcluster)  [unwired: 2 in, 2 out]
                n354 = call-poly "SGUI Assign String With Tags.vi"("error in"=w515, "label(s) (empty)"="stat1\nstat2\nstat3", "string (empty)"="<tc=gold><b>TWM server - Reading results...\n\n") -> ("error out"=w514:errorcluster)  [unwired: 7 in, 1 out]
                n355 = call "SGUI Set Control Enabled State By Groups.vi"("error in"=w514, "group name to enable (none)"="busy") -> ("error out"=w510:errorcluster)  [unwired: 8 in, 1 out]
                n356 = local read "session"() -> (w509:T12)
                n357 = control-ref of="server"() -> (w505:refnum<vi>)
                n358 = call "Server Cmd Answer - Get Result.vi"("server event ref"=w505, "error in"=w510, "client request"=w507, "session in"=w509) -> ("error out"=w506:errorcluster, "session out"=w508:T12)  [unwired: 6 in]
                n359 = local write "session"(w508) -> ()
                n360 = call "SGUI Set Control Enabled State By Groups.vi"("error in"=w506, "group name to enable (none)"="ready") -> ("error out"=w511:errorcluster)  [unwired: 8 in, 1 out]
                n361 = call "GUI Set Error and Display Error Status.vi"("error in"=w511) -> ()  [unwired: 4 in]
              }
            }
          }
          frame "Get algorithm info" {
            n362 = case shown="\"Disabled and Grayed Out\"" w519 {
              tunnel: w520 -> [_ w524]
              tunnel: w518 -> [_ w521]
              frame Default {
              }
              frame "Disabled and Grayed Out" {
                n363 = invoke on="error" class="Clust (strict)" method="Reinit To Default"(error in=w521) -> (error out=w532:errorcluster)  [unwired: 2 in, 2 out]
                n364 = call-poly "SGUI Assign String With Tags.vi"("error in"=w532, "label(s) (empty)"="stat1\nstat2\nstat3", "string (empty)"="<tc=gold><b>TWM server - Get algorithm info...\n\n") -> ("error out"=w531:errorcluster)  [unwired: 7 in, 1 out]
                n365 = call "SGUI Set Control Enabled State By Groups.vi"("error in"=w531, "group name to enable (none)"="busy") -> ("error out"=w527:errorcluster)  [unwired: 8 in, 1 out]
                n366 = local read "session"() -> (w526:T12)
                n367 = control-ref of="server"() -> (w522:refnum<vi>)
                n368 = call "Server Cmd Answer - Get Algorithm Info.vi"("server event ref"=w522, "error in"=w527, "client request"=w524, "session in"=w526) -> ("error out"=w523:errorcluster, "session out"=w525:T12)  [unwired: 6 in]
                n369 = local write "session"(w525) -> ()
                n370 = call "SGUI Set Control Enabled State By Groups.vi"("error in"=w523, "group name to enable (none)"="ready") -> ("error out"=w528:errorcluster)  [unwired: 8 in, 1 out]
                n371 = call "GUI Set Error and Display Error Status.vi"("error in"=w528) -> ()  [unwired: 4 in]
              }
            }
          }
        }
      }
    }
  }
